vi "Virbmain.vi"(0 "Channel 4":T9={" frequency 1"=20, "signal type 1"=enum."Sine Wave", "amplitude 1"=2.0, "offset"=0.0, "phase"=0.0} {"phase" format="%.2p"; "offset" format="%0.2p"; "amplitude 1" format="%0.2p"}, 1 "Channel 3":T9={" frequency 1"=20, "signal type 1"=enum."Sine Wave", "amplitude 1"=2.0, "offset"=0.0, "phase"=0.0} {"phase" format="%.2p"; "offset" format="%0.2p"; "amplitude 1" format="%0.2p"}, 2 "Channel 2":T9={" frequency 1"=20, "signal type 1"=enum."Sine Wave", "amplitude 1"=2.0, "offset"=0.0, "phase"=0.0} {"phase" format="%.2p"; "offset" format="%0.2p"; "amplitude 1" format="%0.2p"}, 3 "Channel 1":T9={" frequency 1"=20, "signal type 1"=enum."Sine Wave", "amplitude 1"=2.0, "offset"=0.0, "phase"=0.0} {"phase" format="%.2p"; "offset" format="%0.2p"; "amplitude 1" format="%0.2p"}, 4 "Time(ms)":i32, 5 "Model List":i32(listbox), 6 "Play Button":bool, 7 "Project Name":string, 9 "OK Button":bool, 10 "Remove Project":bool, 11 "Add Project":bool) -> ()   [LabVIEW 2015]
uses:
  Typedef/Test_State.ctl
  Typedef/State.ctl
  Typedef/Data.ctl
  Typedef/Timer State.ctl
  <vilib>/Utility/xml.llb/Read From XML File(string).vi
  <vilib>/Utility/xml.llb/Write to XML File(string).vi
  <vilib>/measure/NI_MABase.lvlib
panel:
  out "TCP connect":bool
  in  "Right":T1={"Channel 1"={" frequency 1"=25, "signal type 1"=enum."Sine Wave", "amplitude 1"=2.0, "offset"=0.0, "phase"=0.0}, "Channel 2"={" frequency 1"=0, "signal type 1"=enum."Sine Wave", "amplitude 1"=0, "offset"=0.0, "phase"=0.0}, "Channel 3"={" frequency 1"=25, "signal type 1"=enum."Sine Wave", "amplitude 1"=2.0, "offset"=0.0, "phase"=0}, "Channel 4"={" frequency 1"=25, "signal type 1"=enum."Sine Wave", "amplitude 1"=2.0, "offset"=0.0, "phase"=0}}
  in  "Back":T2={"Channel 1"={" frequency 1"=0, "signal type 1"=enum."Sine Wave", "amplitude 1"=0, "offset"=0.0, "phase"=0.0}, "Channel 2"={" frequency 1"=25, "signal type 1"=enum."Sine Wave", "amplitude 1"=2.0, "offset"=0.0, "phase"=0.0}, "Channel 3"={" frequency 1"=25, "signal type 1"=enum."Sine Wave", "amplitude 1"=2.0, "offset"=0, "phase"=0}, "Channel 4"={" frequency 1"=25, "signal type 1"=enum."Sine Wave", "amplitude 1"=2.0, "offset"=0.0, "phase"=0}}
  in  "Left":T3={"Channel 1"={" frequency 1"=25, "signal type 1"=enum."Sine Wave", "amplitude 1"=2.0, "offset"=0, "phase"=0.0}, "Channel 2"={" frequency 1"=25, "signal type 1"=enum."Sine Wave", "amplitude 1"=2.0, "offset"=0, "phase"=0}, "Channel 3"={" frequency 1"=25, "signal type 1"=enum."Sine Wave", "amplitude 1"=2.0, "offset"=0, "phase"=0}, "Channel 4"={" frequency 1"=0, "signal type 1"=enum."Sine Wave", "amplitude 1"=0, "offset"=0, "phase"=0.0}}
  in  "Front":T4={"Channel 1"={" frequency 1"=25, "signal type 1"=enum."Sine Wave", "amplitude 1"=2.0, "offset"=0.0, "phase"=0.0}, "Channel 2"={" frequency 1"=25, "signal type 1"=enum."Sine Wave", "amplitude 1"=2.0, "offset"=0.0, "phase"=0}, "Channel 3"={" frequency 1"=0, "signal type 1"=enum."Sine Wave", "amplitude 1"=0, "offset"=0.0, "phase"=0.0}, "Channel 4"={" frequency 1"=25, "signal type 1"=enum."Sine Wave", "amplitude 1"=2.0, "offset"=0.0, "phase"=0}}
  in  "Center":T5={"Channel 1"={" frequency 1"=25, "signal type 1"=enum."Sine Wave", "amplitude 1"=1.25, "offset"=0, "phase"=0.0}, "Channel 2"={" frequency 1"=25, "signal type 1"=enum."Sine Wave", "amplitude 1"=1.25, "offset"=0, "phase"=90}, "Channel 3"={" frequency 1"=25, "signal type 1"=enum."Sine Wave", "amplitude 1"=1.25, "offset"=0, "phase"=180}, "Channel 4"={" frequency 1"=25, "signal type 1"=enum."Sine Wave", "amplitude 1"=1.25, "offset"=0, "phase"=270}}
  in  "Bump":T6={"Channel 1"={" frequency 1"=25, "signal type 1"=enum."Sine Wave", "amplitude 1"=2.0, "offset"=0, "phase"=0.0}, "Channel 2"={" frequency 1"=25, "signal type 1"=enum."Sine Wave", "amplitude 1"=2.0, "offset"=0, "phase"=0.0}, "Channel 3"={" frequency 1"=25, "signal type 1"=enum."Sine Wave", "amplitude 1"=2.0, "offset"=0, "phase"=0.0}, "Channel 4"={" frequency 1"=25, "signal type 1"=enum."Sine Wave", "amplitude 1"=2.0, "offset"=0, "phase"=0.0}}
  out "Test State":T7
  out "Testing?":bool
  out "Test Setting":waveform(dbl)[](array[waveform])
  out "DataTable":T8(array[cluster])
  in  "Tab Control":enum32{"Main", "Project", "Set"}(tab)
  in  "Setting(Main)":bool
  in  "Project(Main)":bool
  out "Running":bool
  out "Channel 4 Wave (Main)":waveform(dbl)(graph)
  out "Channel 3 Wave (Main)":waveform(dbl)(graph)
  out "Channel 2 Wave (Main)":waveform(dbl)(graph)
  out "Channel 1 Wave (Main)":waveform(dbl)(graph)
  in  "Stop Button":bool
  in  "Center":bool
  in  "Bump":bool
  in  "Rightward":bool
  in  "Leftward":bool
  in  "Backward":bool
  in  "Frontward":bool
  out "Project":string
  in  "Exit Button":bool
  in  "Project List":i32(listbox)
  in  "Main(Project)":bool
  in  "Setting(Project)":bool
  out "Test Time":dbl
  in  "Save Button":bool
  in  "Remove":bool
  in  "Add":bool
  out "Channel 4 Wave":waveform(dbl)(graph)
  out "Channel 3 Wave":waveform(dbl)(graph)
  out "Channel 2 Wave":waveform(dbl)(graph)
  out "Channel 1 Wave":waveform(dbl)(graph)
  out "Testing":bool
  in  "Project(Setting)":bool
  in  "Main(Setting)":bool
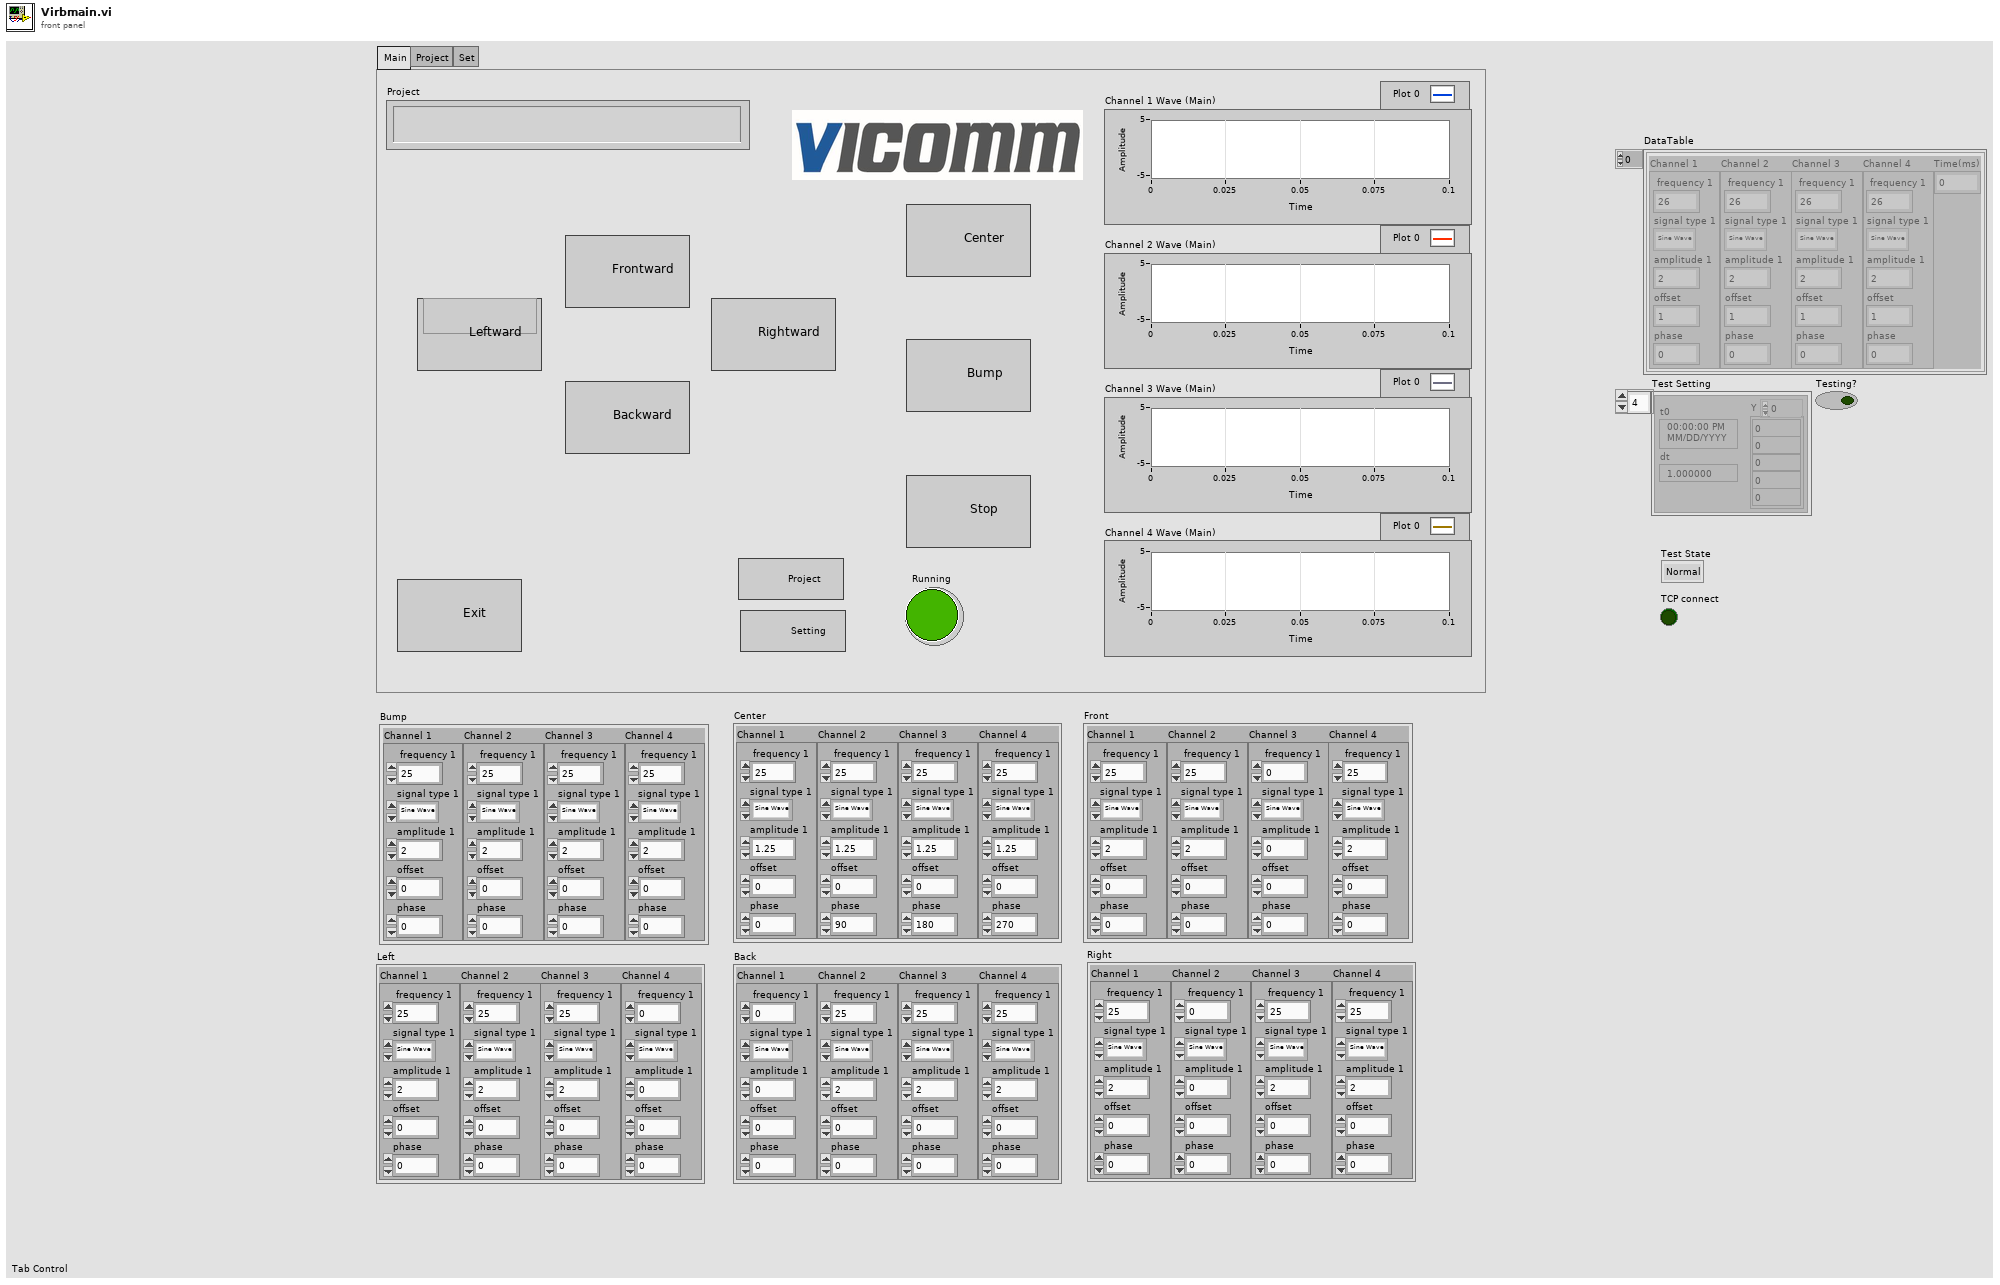
[diagram p1: front panel]
types:
  T1 = cluster{"Channel 1":cluster{" frequency 1":i32, "signal type 1":enum16{"Sine Wave", "Triangle Wave", "Square Wave", "Sawtooth Wave"}, "amplitude 1":dbl, "offset":dbl, "phase":dbl}, "Channel 2":cluster{" frequency 1":i32, "signal type 1":enum16{"Sine Wave", "Triangle Wave", "Square Wave", "Sawtooth Wave"}, "amplitude 1":i32, "offset":dbl, "phase":dbl}, "Channel 3":cluster{" frequency 1":i32, "signal type 1":enum16{"Sine Wave", "Triangle Wave", "Square Wave", "Sawtooth Wave"}, "amplitude 1":dbl, "offset":dbl, "phase":i32}, "Channel 4":cluster{" frequency 1":i32, "signal type 1":enum16{"Sine Wave", "Triangle Wave", "Square Wave", "Sawtooth Wave"}, "amplitude 1":dbl, "offset":dbl, "phase":i32}}
  T2 = cluster{"Channel 1":cluster{" frequency 1":i32, "signal type 1":enum16{"Sine Wave", "Triangle Wave", "Square Wave", "Sawtooth Wave"}, "amplitude 1":i32, "offset":dbl, "phase":dbl}, "Channel 2":cluster{" frequency 1":i32, "signal type 1":enum16{"Sine Wave", "Triangle Wave", "Square Wave", "Sawtooth Wave"}, "amplitude 1":dbl, "offset":dbl, "phase":dbl}, "Channel 3":cluster{" frequency 1":i32, "signal type 1":enum16{"Sine Wave", "Triangle Wave", "Square Wave", "Sawtooth Wave"}, "amplitude 1":dbl, "offset":i32, "phase":i32}, "Channel 4":cluster{" frequency 1":i32, "signal type 1":enum16{"Sine Wave", "Triangle Wave", "Square Wave", "Sawtooth Wave"}, "amplitude 1":dbl, "offset":dbl, "phase":i32}}
  T3 = cluster{"Channel 1":cluster{" frequency 1":i32, "signal type 1":enum16{"Sine Wave", "Triangle Wave", "Square Wave", "Sawtooth Wave"}, "amplitude 1":dbl, "offset":i32, "phase":dbl}, "Channel 2":cluster{" frequency 1":i32, "signal type 1":enum16{"Sine Wave", "Triangle Wave", "Square Wave", "Sawtooth Wave"}, "amplitude 1":dbl, "offset":i32, "phase":i32}, "Channel 3":cluster{" frequency 1":i32, "signal type 1":enum16{"Sine Wave", "Triangle Wave", "Square Wave", "Sawtooth Wave"}, "amplitude 1":dbl, "offset":i32, "phase":i32}, "Channel 4":cluster{" frequency 1":i32, "signal type 1":enum16{"Sine Wave", "Triangle Wave", "Square Wave", "Sawtooth Wave"}, "amplitude 1":i32, "offset":i32, "phase":dbl}}
  T4 = cluster{"Channel 1":cluster{" frequency 1":i32, "signal type 1":enum16{"Sine Wave", "Triangle Wave", "Square Wave", "Sawtooth Wave"}, "amplitude 1":dbl, "offset":dbl, "phase":dbl}, "Channel 2":cluster{" frequency 1":i32, "signal type 1":enum16{"Sine Wave", "Triangle Wave", "Square Wave", "Sawtooth Wave"}, "amplitude 1":dbl, "offset":dbl, "phase":i32}, "Channel 3":cluster{" frequency 1":i32, "signal type 1":enum16{"Sine Wave", "Triangle Wave", "Square Wave", "Sawtooth Wave"}, "amplitude 1":i32, "offset":dbl, "phase":dbl}, "Channel 4":cluster{" frequency 1":i32, "signal type 1":enum16{"Sine Wave", "Triangle Wave", "Square Wave", "Sawtooth Wave"}, "amplitude 1":dbl, "offset":dbl, "phase":i32}}
  T5 = cluster{"Channel 1":cluster{" frequency 1":i32, "signal type 1":enum16{"Sine Wave", "Triangle Wave", "Square Wave", "Sawtooth Wave"}, "amplitude 1":dbl, "offset":i32, "phase":dbl}, "Channel 2":cluster{" frequency 1":i32, "signal type 1":enum16{"Sine Wave", "Triangle Wave", "Square Wave", "Sawtooth Wave"}, "amplitude 1":dbl, "offset":i32, "phase":i32}, "Channel 3":cluster{" frequency 1":i32, "signal type 1":enum16{"Sine Wave", "Triangle Wave", "Square Wave", "Sawtooth Wave"}, "amplitude 1":dbl, "offset":i32, "phase":i32}, "Channel 4":cluster{" frequency 1":i32, "signal type 1":enum16{"Sine Wave", "Triangle Wave", "Square Wave", "Sawtooth Wave"}, "amplitude 1":dbl, "offset":i32, "phase":i32}}
  T6 = cluster{"Channel 1":cluster{" frequency 1":i32, "signal type 1":enum16{"Sine Wave", "Triangle Wave", "Square Wave", "Sawtooth Wave"}, "amplitude 1":dbl, "offset":i32, "phase":dbl}, "Channel 2":cluster{" frequency 1":i32, "signal type 1":enum16{"Sine Wave", "Triangle Wave", "Square Wave", "Sawtooth Wave"}, "amplitude 1":dbl, "offset":i32, "phase":dbl}, "Channel 3":cluster{" frequency 1":i32, "signal type 1":enum16{"Sine Wave", "Triangle Wave", "Square Wave", "Sawtooth Wave"}, "amplitude 1":dbl, "offset":i32, "phase":dbl}, "Channel 4":cluster{" frequency 1":i32, "signal type 1":enum16{"Sine Wave", "Triangle Wave", "Square Wave", "Sawtooth Wave"}, "amplitude 1":dbl, "offset":i32, "phase":dbl}}
  T7 = typedef "Test_State.ctl" = enum16{"Normal", "Bump", "Center"}
  T8 = cluster{"Channel 1":cluster{" frequency 1":u32, "signal type 1":enum16{"Sine Wave", "Triangle Wave", "Square Wave", "Sawtooth Wave"}, "amplitude 1":dbl, "offset":dbl, "phase":dbl}, "Channel 2":cluster{" frequency 1":u32, "signal type 1":enum16{"Sine Wave", "Triangle Wave", "Square Wave", "Sawtooth Wave"}, "amplitude 1":dbl, "offset":dbl, "phase":dbl}, "Channel 3":cluster{" frequency 1":u32, "signal type 1":enum16{"Sine Wave", "Triangle Wave", "Square Wave", "Sawtooth Wave"}, "amplitude 1":dbl, "offset":dbl, "phase":dbl}, "Channel 4":cluster{" frequency 1":u32, "signal type 1":enum16{"Sine Wave", "Triangle Wave", "Square Wave", "Sawtooth Wave"}, "amplitude 1":dbl, "offset":dbl, "phase":dbl}, "Time(ms)":i32}[]
  T9 = cluster{" frequency 1":u32, "signal type 1":enum16{"Sine Wave", "Triangle Wave", "Square Wave", "Sawtooth Wave"}, "amplitude 1":dbl, "offset":dbl, "phase":dbl}
  T10 = typedef "Data.ctl" = cluster{"Channel Table":cluster{"Channel 1":cluster{" frequency 1":u32, "signal type 1":enum16{"Sine Wave", "Triangle Wave", "Square Wave", "Sawtooth Wave"}, "amplitude 1":dbl, "offset":dbl, "phase":dbl}, "Channel 2":cluster{" frequency 1":u32, "signal type 1":enum16{"Sine Wave", "Triangle Wave", "Square Wave", "Sawtooth Wave"}, "amplitude 1":dbl, "offset":dbl, "phase":dbl}, "Channel 3":cluster{" frequency 1":u32, "signal type 1":enum16{"Sine Wave", "Triangle Wave", "Square Wave", "Sawtooth Wave"}, "amplitude 1":dbl, "offset":dbl, "phase":dbl}, "Channel 4":cluster{" frequency 1":u32, "signal type 1":enum16{"Sine Wave", "Triangle Wave", "Square Wave", "Sawtooth Wave"}, "amplitude 1":dbl, "offset":dbl, "phase":dbl}, "Time(ms)":i32}[], "Model List name":string[], "Channel 1 Wave":waveform(dbl), "Channel 2 Wave":waveform(dbl), "Channel 3 Wave":waveform(dbl), "Channel 4 Wave":waveform(dbl), "Testing":bool, "Set Time":i32, "Elapse Time":dbl, "Channel 1":cluster{" frequency 1":u32, "signal type 1":enum16{"Sine Wave", "Triangle Wave", "Square Wave", "Sawtooth Wave"}, "amplitude 1":dbl, "offset":dbl, "phase":dbl}, "Channel 2":cluster{" frequency 1":u32, "signal type 1":enum16{"Sine Wave", "Triangle Wave", "Square Wave", "Sawtooth Wave"}, "amplitude 1":dbl, "offset":dbl, "phase":dbl}, "Channel 3":cluster{" frequency 1":u32, "signal type 1":enum16{"Sine Wave", "Triangle Wave", "Square Wave", "Sawtooth Wave"}, "amplitude 1":dbl, "offset":dbl, "phase":dbl}, "Channel 4":cluster{" frequency 1":u32, "signal type 1":enum16{"Sine Wave", "Triangle Wave", "Square Wave", "Sawtooth Wave"}, "amplitude 1":dbl, "offset":dbl, "phase":dbl}, "ModelList Num":i32, "Stop":bool, "Button":bool, "Button Time":i32, "Elapsed ?":bool, "Channel 1 Wave (Main)":waveform(dbl), "Channel 2 Wave (Main)":waveform(dbl), "Channel 3 Wave (Main)":waveform(dbl), "Channel 4 Wave (Main)":waveform(dbl), "Project List name":string[], "Project Name":string, "Project Path":path, "ProjectList Num":i32, "Project Name(Set)":string}
  T11 = enum16{"Standard", "Buffered", "CRLF", "Immediate"}
  T12 = typedef "State.ctl" = enum16{"Initalize", "Idle", "Update", "Channel1", "Channel2", "Channel3", "Channel4", "ModelList", "Add", "Remove", "Set Time", "Test", "Start Time", "Check Time", "Save", "Frontward", "Leftward", "Backward", "Rightward", "Stop", "Center", "Bump", "Add Project", "Remove Project", "Project List", "Project Name", "Project OK", "Exit"}
  T13 = typedef "Timer State.ctl" = enum16{"Start", "Check"}
  T14 = cluster{"State":T12, "Channel 1":cluster{" frequency 1":u32, "signal type 1":enum16{"Sine Wave", "Triangle Wave", "Square Wave", "Sawtooth Wave"}, "amplitude 1":dbl, "offset":dbl, "phase":dbl}}
  T15 = cluster{"State":T12, "Channel 2":cluster{" frequency 1":u32, "signal type 1":enum16{"Sine Wave", "Triangle Wave", "Square Wave", "Sawtooth Wave"}, "amplitude 1":dbl, "offset":dbl, "phase":dbl}}
  T16 = cluster{"State":T12, "Channel 3":cluster{" frequency 1":u32, "signal type 1":enum16{"Sine Wave", "Triangle Wave", "Square Wave", "Sawtooth Wave"}, "amplitude 1":dbl, "offset":dbl, "phase":dbl}}
  T17 = cluster{"State":T12, "Channel 4":cluster{" frequency 1":u32, "signal type 1":enum16{"Sine Wave", "Triangle Wave", "Square Wave", "Sawtooth Wave"}, "amplitude 1":dbl, "offset":dbl, "phase":dbl}}
  T18 = cluster{"DataTable":cluster{"Channel 1":cluster{" frequency 1":u32, "signal type 1":enum16{"Sine Wave", "Triangle Wave", "Square Wave", "Sawtooth Wave"}, "amplitude 1":dbl, "offset":dbl, "phase":dbl}, "Channel 2":cluster{" frequency 1":u32, "signal type 1":enum16{"Sine Wave", "Triangle Wave", "Square Wave", "Sawtooth Wave"}, "amplitude 1":dbl, "offset":dbl, "phase":dbl}, "Channel 3":cluster{" frequency 1":u32, "signal type 1":enum16{"Sine Wave", "Triangle Wave", "Square Wave", "Sawtooth Wave"}, "amplitude 1":dbl, "offset":dbl, "phase":dbl}, "Channel 4":cluster{" frequency 1":u32, "signal type 1":enum16{"Sine Wave", "Triangle Wave", "Square Wave", "Sawtooth Wave"}, "amplitude 1":dbl, "offset":dbl, "phase":dbl}, "Time(ms)":i32}[], "Item Names":string[]}
  T19 = enum16{"Sine Wave", "Triangle Wave", "Square Wave", "Sawtooth Wave"}
  T20 = cluster{"Channel 1":cluster{" frequency 1":u32, "signal type 1":enum16{"Sine Wave", "Triangle Wave", "Square Wave", "Sawtooth Wave"}, "amplitude 1":dbl, "offset":dbl, "phase":dbl}, "Channel 2":cluster{" frequency 1":u32, "signal type 1":enum16{"Sine Wave", "Triangle Wave", "Square Wave", "Sawtooth Wave"}, "amplitude 1":dbl, "offset":dbl, "phase":dbl}, "Channel 3":cluster{" frequency 1":u32, "signal type 1":enum16{"Sine Wave", "Triangle Wave", "Square Wave", "Sawtooth Wave"}, "amplitude 1":dbl, "offset":dbl, "phase":dbl}, "Channel 4":cluster{" frequency 1":u32, "signal type 1":enum16{"Sine Wave", "Triangle Wave", "Square Wave", "Sawtooth Wave"}, "amplitude 1":dbl, "offset":dbl, "phase":dbl}, "Time(ms)":i32}
  T21 = cluster{" frequency 1":u32, "signal type 1":enum16{"Sine Wave", "Triangle Wave", "Square Wave", "Sawtooth Wave"}, "amplitude 1":dbl, "offset":dbl, "phase":dbl}[]
  T22 = cluster{"Channel 1":cluster{" frequency 1":u32, "signal type 1":enum16{"Sine Wave", "Triangle Wave", "Square Wave", "Sawtooth Wave"}, "amplitude 1":dbl, "offset":dbl, "phase":dbl}, "Channel 2":cluster{" frequency 1":u32, "signal type 1":enum16{"Sine Wave", "Triangle Wave", "Square Wave", "Sawtooth Wave"}, "amplitude 1":dbl, "offset":dbl, "phase":dbl}, "Channel 3":cluster{" frequency 1":u32, "signal type 1":enum16{"Sine Wave", "Triangle Wave", "Square Wave", "Sawtooth Wave"}, "amplitude 1":dbl, "offset":dbl, "phase":dbl}, "Channel 4":cluster{" frequency 1":u32, "signal type 1":enum16{"Sine Wave", "Triangle Wave", "Square Wave", "Sawtooth Wave"}, "amplitude 1":dbl, "offset":dbl, "phase":dbl}, "Set Time":i32}
  T23 = cluster{"Channel 1":cluster{" frequency 1":u32, "signal type 1":enum16{"Sine Wave", "Triangle Wave", "Square Wave", "Sawtooth Wave"}, "amplitude 1":dbl, "offset":dbl, "phase":dbl}, "Channel 2":cluster{" frequency 1":u32, "signal type 1":enum16{"Sine Wave", "Triangle Wave", "Square Wave", "Sawtooth Wave"}, "amplitude 1":dbl, "offset":dbl, "phase":dbl}, "Channel 3":cluster{" frequency 1":u32, "signal type 1":enum16{"Sine Wave", "Triangle Wave", "Square Wave", "Sawtooth Wave"}, "amplitude 1":dbl, "offset":dbl, "phase":dbl}, "Channel 4":cluster{" frequency 1":u32, "signal type 1":enum16{"Sine Wave", "Triangle Wave", "Square Wave", "Sawtooth Wave"}, "amplitude 1":dbl, "offset":dbl, "phase":dbl}, "Set Time":i32}[]
  T24 = cluster{"Channel Table":cluster{"Channel 1":cluster{" frequency 1":u32, "signal type 1":enum16{"Sine Wave", "Triangle Wave", "Square Wave", "Sawtooth Wave"}, "amplitude 1":dbl, "offset":dbl, "phase":dbl}, "Channel 2":cluster{" frequency 1":u32, "signal type 1":enum16{"Sine Wave", "Triangle Wave", "Square Wave", "Sawtooth Wave"}, "amplitude 1":dbl, "offset":dbl, "phase":dbl}, "Channel 3":cluster{" frequency 1":u32, "signal type 1":enum16{"Sine Wave", "Triangle Wave", "Square Wave", "Sawtooth Wave"}, "amplitude 1":dbl, "offset":dbl, "phase":dbl}, "Channel 4":cluster{" frequency 1":u32, "signal type 1":enum16{"Sine Wave", "Triangle Wave", "Square Wave", "Sawtooth Wave"}, "amplitude 1":dbl, "offset":dbl, "phase":dbl}, "Time(ms)":i32}[], "Model List name":string[]}
  T25 = cluster{" frequency 1":i32, "signal type 1":enum16{"Sine Wave", "Triangle Wave", "Square Wave", "Sawtooth Wave"}, "amplitude 1":dbl, "offset":dbl, "phase":dbl}
  T26 = cluster{" frequency 1":i32, "signal type 1":enum16{"Sine Wave", "Triangle Wave", "Square Wave", "Sawtooth Wave"}, "amplitude 1":dbl, "offset":dbl, "phase":i32}
  T27 = cluster{" frequency 1":i32, "signal type 1":enum16{"Sine Wave", "Triangle Wave", "Square Wave", "Sawtooth Wave"}, "amplitude 1":i32, "offset":dbl, "phase":dbl}
  T28 = cluster{" frequency 1":i32, "signal type 1":enum16{"Sine Wave", "Triangle Wave", "Square Wave", "Sawtooth Wave"}, "amplitude 1":dbl, "offset":dbl, "phase":dbl}[]
  T29 = cluster{" frequency 1":i32, "signal type 1":enum16{"Sine Wave", "Triangle Wave", "Square Wave", "Sawtooth Wave"}, "amplitude 1":dbl, "offset":i32, "phase":dbl}
  T30 = cluster{" frequency 1":i32, "signal type 1":enum16{"Sine Wave", "Triangle Wave", "Square Wave", "Sawtooth Wave"}, "amplitude 1":dbl, "offset":i32, "phase":i32}
  T31 = cluster{" frequency 1":i32, "signal type 1":enum16{"Sine Wave", "Triangle Wave", "Square Wave", "Sawtooth Wave"}, "amplitude 1":i32, "offset":i32, "phase":dbl}
  T32 = cluster{" frequency 1":i32, "signal type 1":enum16{"Sine Wave", "Triangle Wave", "Square Wave", "Sawtooth Wave"}, "amplitude 1":dbl, "offset":i32, "phase":dbl}[]
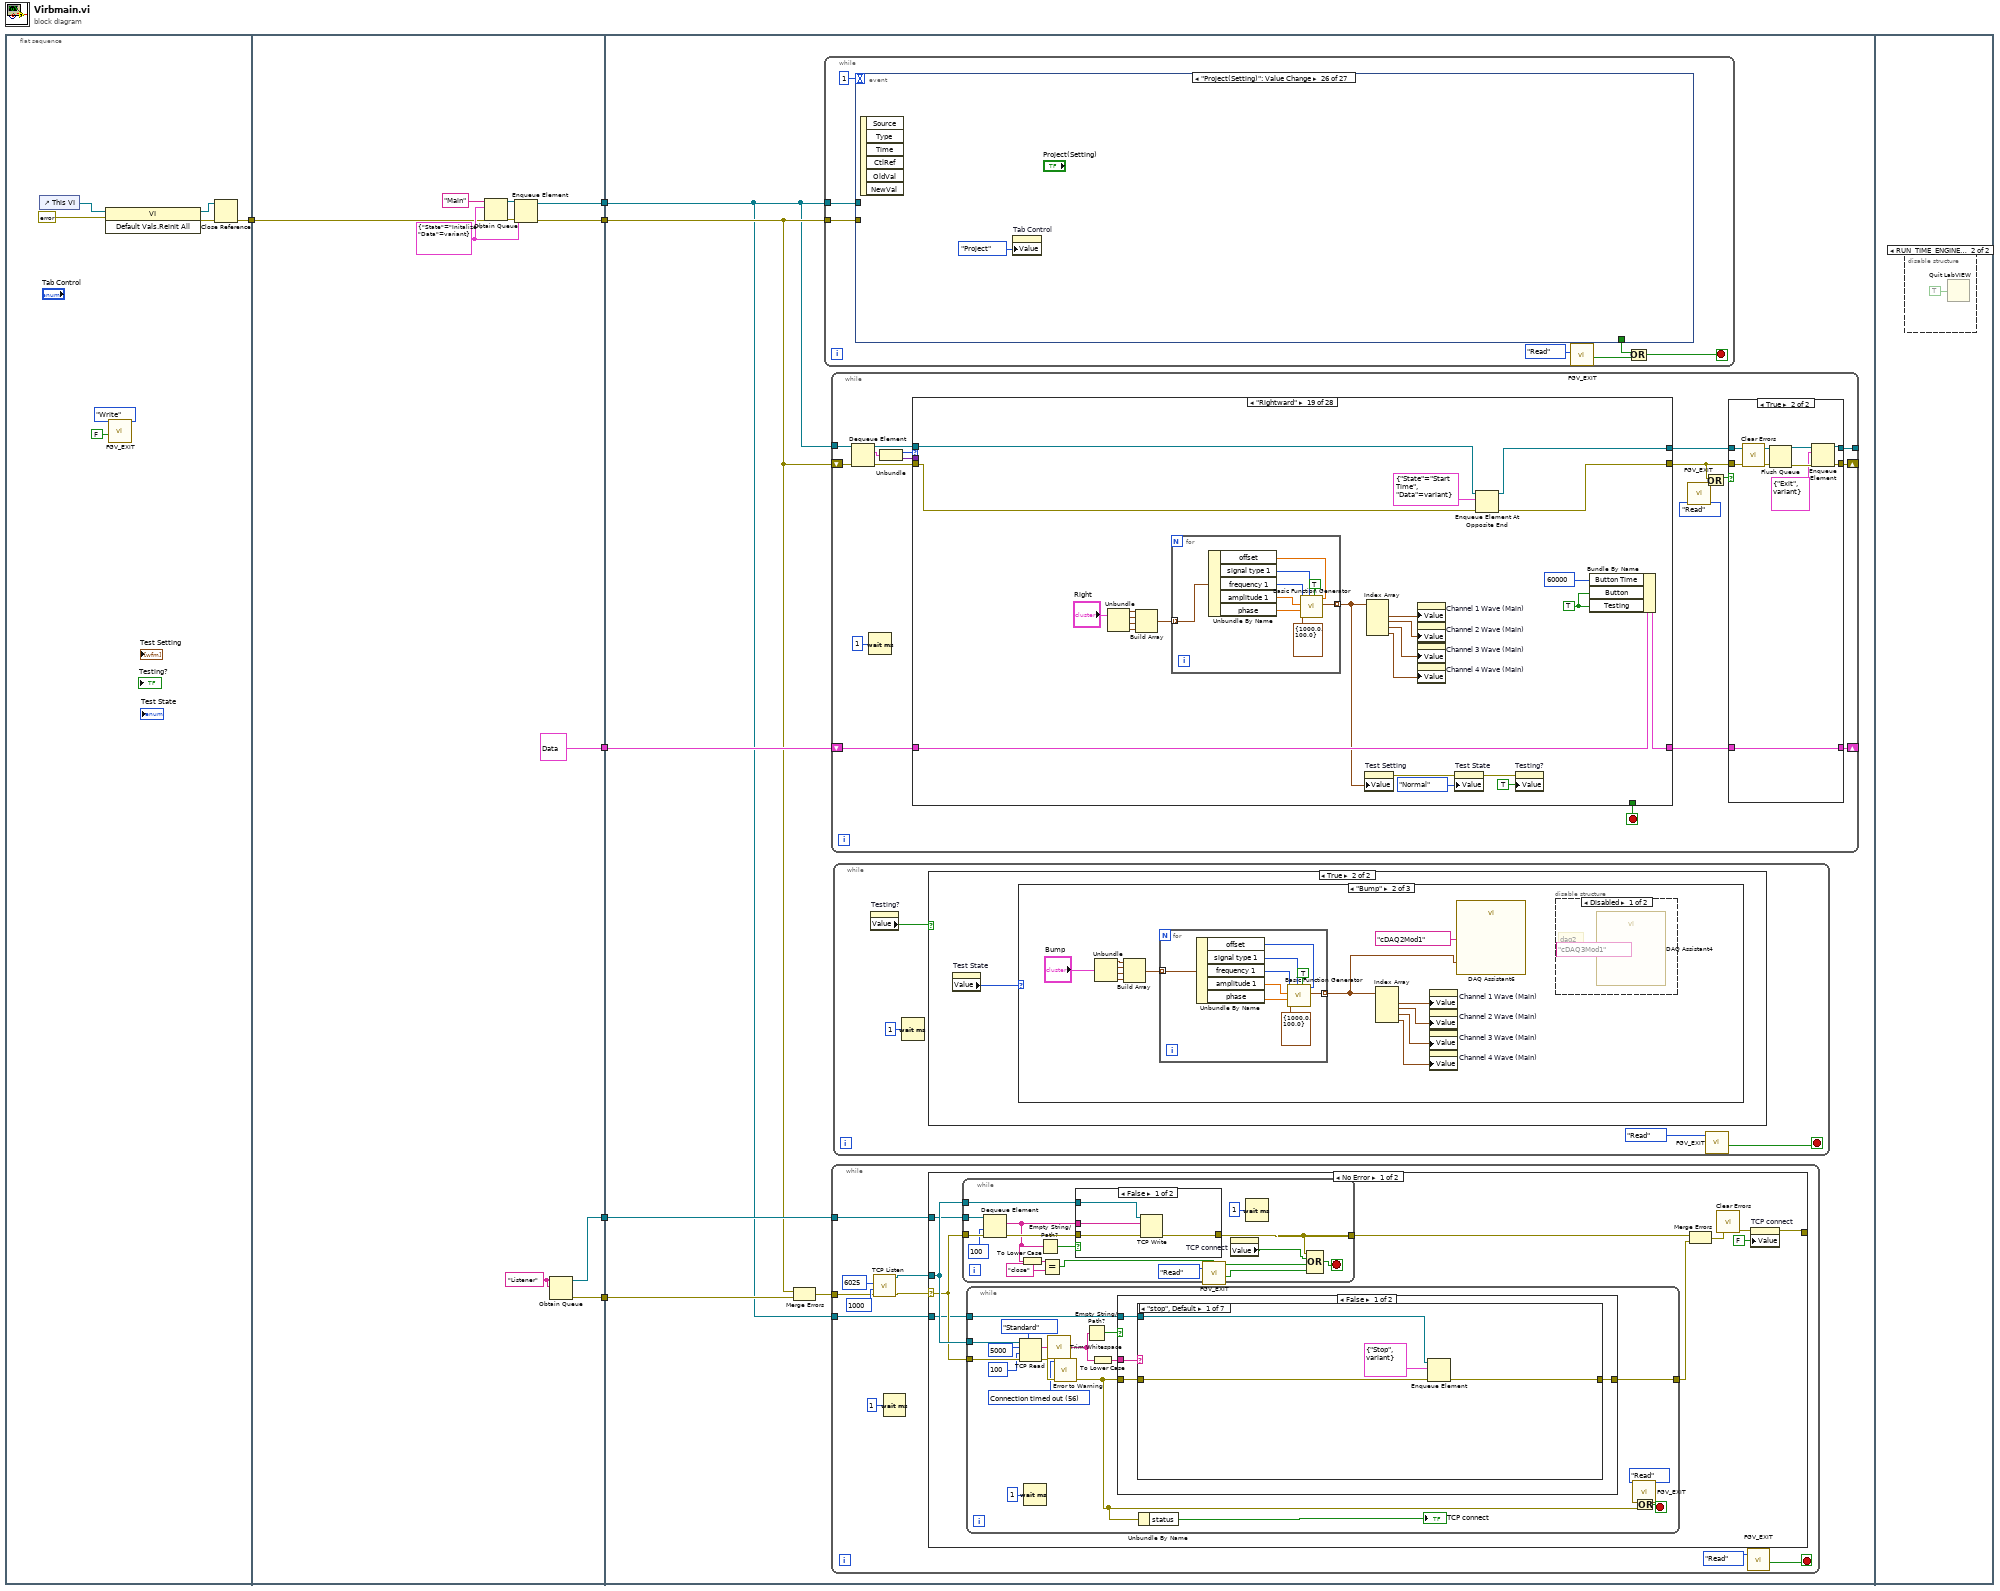
[diagram p0: block diagram]
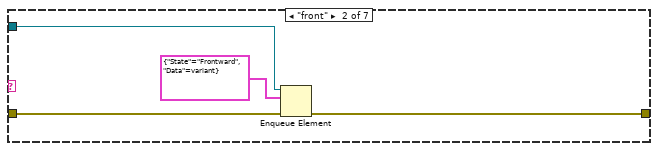
[diagram p2: hidden frame]
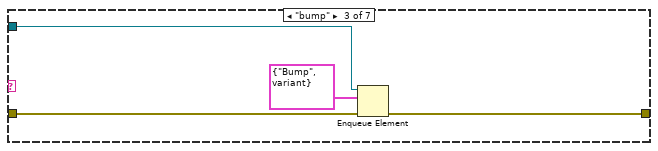
[diagram p3: hidden frame]
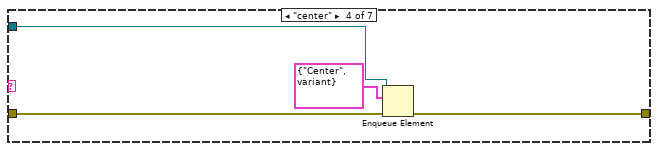
[diagram p4: hidden frame]
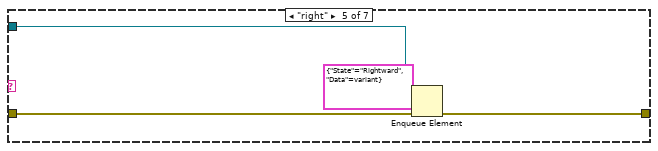
[diagram p5: hidden frame]
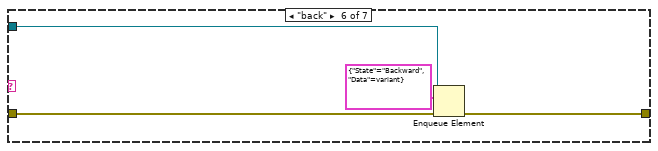
[diagram p6: hidden frame]
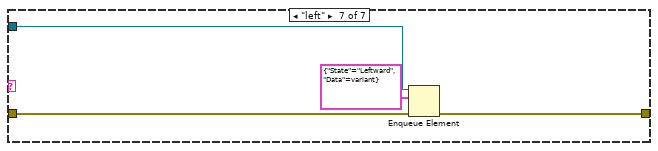
[diagram p7: hidden frame]
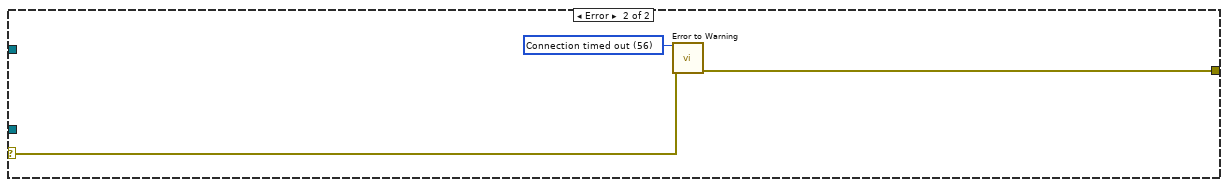
[diagram p10: hidden frame]
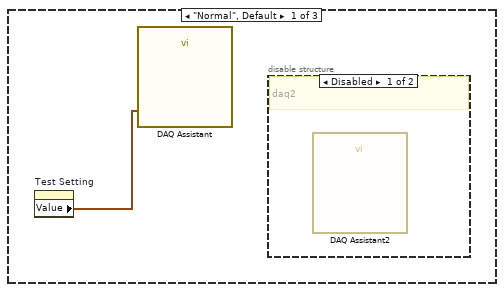
[diagram p12: hidden frame]
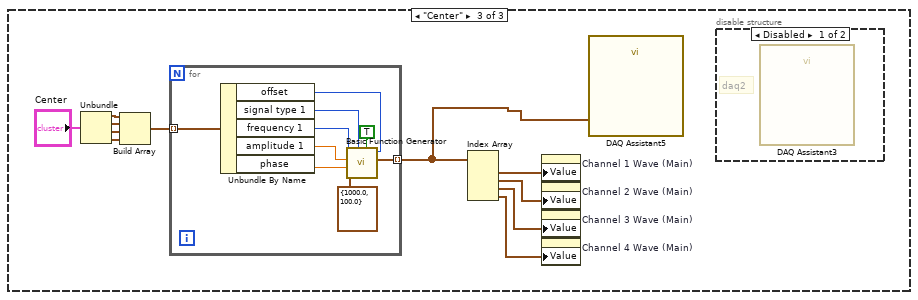
[diagram p15: hidden frame]
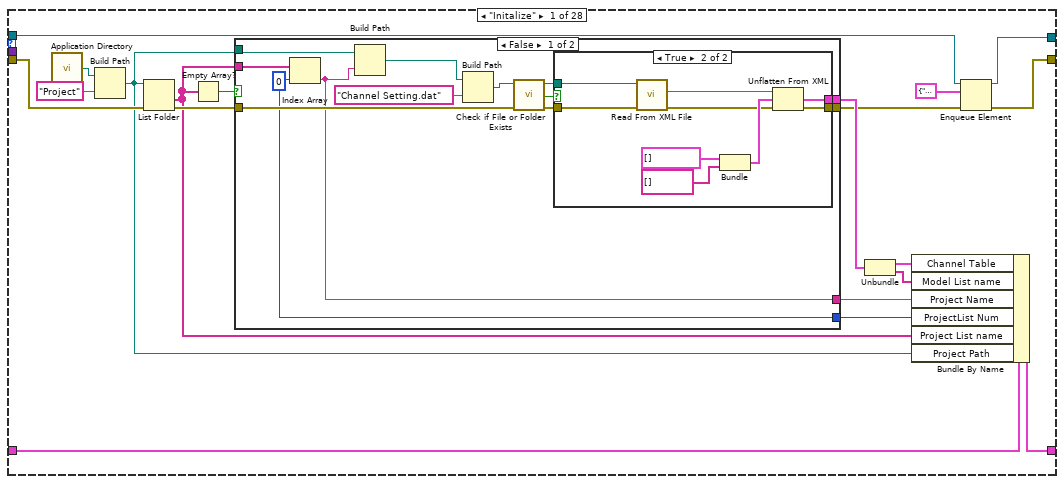
[diagram p18: hidden frame]
diagram:
  n1 = flat-sequence {
    tunnel: [w10] -> w3
    tunnel: [w20] -> w6
    tunnel: [w19] -> w5
    tunnel: [T10 {"Channel Table"=[], "Model List name"=[], "Channel 1 Wave"={"t0"=timestamp(0 s since 1904-01-01), "dt"=1.0, "Y"=[]}, "Channel 2 Wave"={"t0"=timestamp(0 s since 1904-01-01), "dt"=1.0, "Y"=[]}, "Channel 3 Wave"={"t0"=timestamp(0 s since 1904-01-01), "dt"=1.0, "Y"=[]}, "Channel 4 Wave"={"t0"=timestamp(0 s since 1904-01-01), "dt"=1.0, "Y"=[]}, "Testing"=FALSE, "Set Time"=0, "Elapse Time"=0.0, "Channel 1"={" frequency 1"=20, "signal type 1"=enum."Sine Wave", "amplitude 1"=2.0, "offset"=0.0, "phase"=0.0}, "Channel 2"={" frequency 1"=20, "signal type 1"=enum."Sine Wave", "amplitude 1"=2.0, "offset"=0.0, "phase"=0.0}, "Channel 3"={" frequency 1"=20, "signal type 1"=enum."Sine Wave", "amplitude 1"=2.0, "offset"=0.0, "phase"=0.0}, "Channel 4"={" frequency 1"=20, "signal type 1"=enum."Sine Wave", "amplitude 1"=2.0, "offset"=0.0, "phase"=0.0}, "ModelList Num"=0, "Stop"=FALSE, "Button"=FALSE, "Button Time"=0, "Elapsed ?"=FALSE, "Channel 1 Wave (Main)"={"t0"=timestamp(0 s since 1904-01-01), "dt"=1.0, "Y"=[]}, "Channel 2 Wave (Main)"={"t0"=timestamp(0 s since 1904-01-01), "dt"=1.0, "Y"=[]}, "Channel 3 Wave (Main)"={"t0"=timestamp(0 s since 1904-01-01), "dt"=1.0, "Y"=[]}, "Channel 4 Wave (Main)"={"t0"=timestamp(0 s since 1904-01-01), "dt"=1.0, "Y"=[]}, "Project List name"=[], "Project Name"="", "Project Path"=path "", "ProjectList Num"=0, "Project Name(Set)"=""}] -> w4
    tunnel: w3 -> [w17]
    tunnel: [w15] -> w2
    tunnel: [w14] -> w1
    tunnel: w6 -> [w25]
    tunnel: w5 -> [w26]
    tunnel: w4 -> [w30]
    tunnel: w2 -> [w29]
    tunnel: w1 -> [w28]
    frame #0 {
      n2 = control-ref of="This VI"() -> (w13:refnum<vi>)
      n3 = invoke class="VI" method="Default Vals.Reinit All"(reference=w13, error in=errorcluster {"status"=FALSE, "code"=0, "source"=""} ("error in (no error)")) -> (reference out=w11:refnum<vi>, error out=w12:errorcluster)  [unwired: 1 in, 1 out]
      n4 = call "FGV_EXIT.vi"("Function"=enum16{"Read", "Write"}."Write", "EXIT"=FALSE) -> ()  [unwired: 6 in, 1 out]
      n5 = Close Reference(reference=w11, error in (no error)=w12) -> (error out=w10:errorcluster)
    }
    frame #1 {
      w16 = "Listener" ("name (unnamed)")
      w21 = cluster{"State":T12, "Data":variant} {"State"=enum."Initalize", "Data"=variant}
      n6 = Obtain Queue(name (unnamed)="Main", element data type=w21, error in (no error)=w17) -> (queue out=w23:refnum<queue>, error out=w24:errorcluster)  [unwired: 2 in, 1 out]
      n7 = Enqueue Element(queue=w23, element=w21, error in (no error)=w24) -> (queue out=w20:refnum<queue>, error out=w19:errorcluster)  [unwired: 1 in, 1 out]
      n8 = Obtain Queue(name (unnamed)=w16, element data type=w16) -> (queue out=w15:refnum<queue>, error out=w14:errorcluster)  [unwired: 3 in, 1 out]
    }
    frame #2 {
      n9 = Merge Errors(w26, w28) -> (w27:errorcluster)
      n10 = while {
        tunnel: w25 -> [w818]
        tunnel: w26 -> [w817]
        stop <- w815 stop-if-true
        n11 = event shown="[25] \"Project(Setting)\": Value Change" {
          selector: _ -> [_ _ _ _ _ _ _ _ _ _ _ _ _ _ _ _ _ _ _ _ _ _ _ _ _ _ _]
          dyn-events: _ -> [_ _ _ _ _ _ _ _ _ _ _ _ _ _ _ _ _ _ _ _ _ _ _ _ _ _ _]
          timeout: 1 -> [_ _ _ _ _ _ _ _ _ _ _ _ _ _ _ _ _ _ _ _ _ _ _ _ _ _ _]
          tunnel: [_ w821 _ _ _ _ _ _ _ _ _ _ _ _ _ _ _ _ _ _ _ _ _ _ _ _ _] -> w819
          tunnel: w818 -> [_ w825 w829 w834 w840 w872 w875 w878 w881 w884 w887 w890 w893 w896 w899 w902 w905 w910 w915 w919 w921 _ _ _ _ _ _]
          tunnel: w817 -> [_ w826 w828 w835 w839 w873 w876 w879 w882 w885 w888 w891 w894 w897 w900 w903 w906 w911 w916 w918 w922 _ _ _ _ _ _]
          event Timeout {
            n12 = event-data() -> ()  [unwired: 1 in, 3 out]
          }
          event "Exit Button": Value Change {
            w821 = TRUE
            n13 = event-data() -> ()  [unwired: 1 in, 2 out]
            n14 = Flush Queue(queue=w825, error in (no error)=w826) -> (queue out=w823:refnum<queue>, error out=w824:errorcluster)  [unwired: 1 out]
            n15 = Enqueue Element(queue=w823, element=cluster{"State":T12, "Data":variant} {"State"=enum."Exit", "Data"=variant}, error in (no error)=w824) -> ()  [unwired: 1 in, 3 out]
            n16 = call "FGV_EXIT.vi"("Function"=enum16{"Read", "Write"}."Write", "EXIT"=w821) -> ()  [unwired: 6 in, 1 out]
          }
          event "Play Button": Value Change {
            n17 = event-data() -> ()  [unwired: 1 in, 6 out]
            n18 = Enqueue Element(queue=w829, element=cluster{"State":T12, "Data":variant} {"State"=enum."Test", "Data"=variant}, error in (no error)=w828) -> ()  [unwired: 1 in, 3 out]
          }
          event "Time(ms)": Value Change {
            n19 = event-data() -> ()  [unwired: 1 in, 1 out]
            n20 = Bundle(cluster=cluster{"State":T12, "Data":variant} {"State"=enum."Initalize", "Data"=variant}, "State"=State."Set Time", "Data"="Time(ms)") -> (w832:cluster{"State":T12, "Data":variant})
            n21 = Enqueue Element(queue=w834, element=w832, error in (no error)=w835) -> ()  [unwired: 1 in, 3 out]
          }
          event "Channel 1", "Channel 2", "Channel 4", "Channel 3": Value Change {
            n22 = event-data() -> ("CtlRef"=w845:refnum<vi>)  [unwired: 1 in]
            n23 = property class="Clust (strict)"(reference=w845) -> ("Label.Text"=w844:string)  [unwired: 1 in, 2 out]
            n24 = Match Pattern(string=w844, regular expression="Channel") -> (after substring=w842:string)  [unwired: 1 in, 3 out]
            n25 = Decimal String To Number(string=w842) -> (number=w841:i32)  [unwired: 2 in, 1 out]
            n26 = case shown="4" w841 {
              tunnel: w840 -> [w848 w852 w857 w862 w867]
              tunnel: w839 -> [w847 w853 w858 w863 w868]
              tunnel: [w847 w853 w858 w863 w868] -> w838
              tunnel: [w848 w852 w857 w862 w867] -> w837
              tunnel: [cluster{"State":T12, "Data":variant} {"State"=enum."Update", "Data"=variant} w850 w856 w860 w866] -> w836
              frame 0, Default {
              }
              frame 1 {
                n27 = Bundle("State"=State."Channel1", "Channel 1"="Channel 1") -> (w850:T14)  [unwired: 1 in]
              }
              frame 2 {
                n28 = Bundle("State"=State."Channel2", "Channel 2"="Channel 2") -> (w856:T15)  [unwired: 1 in]
              }
              frame 3 {
                n29 = Bundle("State"=State."Channel3", "Channel 3"="Channel 3") -> (w860:T16)  [unwired: 1 in]
              }
              frame 4 {
                n30 = Bundle("State"=State."Channel4", "Channel 4"="Channel 4") -> (w866:T17)  [unwired: 1 in]
              }
            }
            n31 = Enqueue Element(queue=w837, element=w836, error in (no error)=w838) -> ()  [unwired: 1 in, 3 out]
          }
          event "Model List": Value Change {
            n32 = event-data() -> ("NewVal"=w869:i32)  [unwired: 1 in]
            n33 = Bundle By Name(cluster=cluster{"State":T12, "Data":variant} {"State"=enum."ModelList", "Data"=variant}, "Data"=w869) -> (w871:cluster{"State":T12, "Data":variant})
            n34 = Enqueue Element(queue=w872, element=w871, error in (no error)=w873) -> ()  [unwired: 1 in, 3 out]
          }
          event "Add": Value Change {
            n35 = event-data() -> ()  [unwired: 1 in, 1 out]
            n36 = Enqueue Element(queue=w875, element=cluster{"State":T12, "Data":variant} {"State"=enum."Add", "Data"=variant}, error in (no error)=w876) -> ()  [unwired: 1 in, 3 out]
          }
          event "Remove": Value Change {
            n37 = event-data() -> ()  [unwired: 1 in, 2 out]
            n38 = Enqueue Element(queue=w878, element=cluster{"State":T12, "Data":variant} {"State"=enum."Remove", "Data"=variant}, error in (no error)=w879) -> ()  [unwired: 1 in, 3 out]
          }
          event "Save Button": Value Change {
            n39 = event-data() -> ()  [unwired: 1 in, 2 out]
            n40 = Enqueue Element(queue=w881, element=cluster{"State":T12, "Data":variant} {"State"=enum."Save", "Data"=variant}, error in (no error)=w882) -> ()  [unwired: 1 in, 3 out]
          }
          event "Frontward": Value Change {
            n41 = event-data() -> ()  [unwired: 1 in, 2 out]
            n42 = Enqueue Element(queue=w884, element=cluster{"State":T12, "Data":variant} {"State"=enum."Frontward", "Data"=variant}, error in (no error)=w885) -> ()  [unwired: 1 in, 3 out]
          }
          event "Leftward": Value Change {
            n43 = event-data() -> ()  [unwired: 1 in, 2 out]
            n44 = Enqueue Element(queue=w887, element=cluster{"State":T12, "Data":variant} {"State"=enum."Leftward", "Data"=variant}, error in (no error)=w888) -> ()  [unwired: 1 in, 3 out]
          }
          event "Backward": Value Change {
            n45 = event-data() -> ()  [unwired: 1 in, 2 out]
            n46 = Enqueue Element(queue=w890, element=cluster{"State":T12, "Data":variant} {"State"=enum."Backward", "Data"=variant}, error in (no error)=w891) -> ()  [unwired: 1 in, 3 out]
          }
          event "Rightward": Value Change {
            n47 = event-data() -> ()  [unwired: 1 in, 2 out]
            n48 = Enqueue Element(queue=w893, element=cluster{"State":T12, "Data":variant} {"State"=enum."Rightward", "Data"=variant}, error in (no error)=w894) -> ()  [unwired: 1 in, 3 out]
          }
          event "Center": Value Change {
            n49 = event-data() -> ()  [unwired: 1 in, 6 out]
            n50 = Enqueue Element(queue=w896, element=cluster{"State":T12, "Data":variant} {"State"=enum."Center", "Data"=variant}, error in (no error)=w897) -> ()  [unwired: 1 in, 3 out]
          }
          event "Bump": Value Change {
            n51 = event-data() -> ()  [unwired: 1 in, 6 out]
            n52 = Enqueue Element(queue=w899, element=cluster{"State":T12, "Data":variant} {"State"=enum."Bump", "Data"=variant}, error in (no error)=w900) -> ()  [unwired: 1 in, 3 out]
          }
          event "Add Project": Value Change {
            n53 = event-data() -> ()  [unwired: 1 in, 6 out]
            n54 = Enqueue Element(queue=w902, element=cluster{"State":T12, "Data":variant} {"State"=enum."Add Project", "Data"=variant}, error in (no error)=w903) -> ()  [unwired: 1 in, 3 out]
          }
          event "Remove Project": Value Change {
            n55 = event-data() -> ()  [unwired: 1 in, 6 out]
            n56 = Enqueue Element(queue=w905, element=cluster{"State":T12, "Data":variant} {"State"=enum."Remove Project", "Data"=variant}, error in (no error)=w906) -> ()  [unwired: 1 in, 3 out]
          }
          event "Project Name": Value Change {
            n57 = event-data() -> ("NewVal"=w907:string)  [unwired: 1 in]
            n58 = Bundle By Name(cluster=cluster{"State":T12, "Data":variant} {"State"=enum."Project Name", "Data"=variant}, "Data"=w907) -> (w908:cluster{"State":T12, "Data":variant})
            n59 = Enqueue Element(queue=w910, element=w908, error in (no error)=w911) -> ()  [unwired: 1 in, 3 out]
          }
          event "Project List": Value Change {
            n60 = event-data() -> ("NewVal"=w912:i32)  [unwired: 1 in, 5 out]
            n61 = Bundle By Name(cluster=cluster{"State":T12, "Data":variant} {"State"=enum."Project List", "Data"=variant}, "Data"=w912) -> (w913:cluster{"State":T12, "Data":variant})
            n62 = Enqueue Element(queue=w915, element=w913, error in (no error)=w916) -> ()  [unwired: 1 in, 3 out]
          }
          event "OK Button": Value Change {
            n63 = event-data() -> ()  [unwired: 1 in, 6 out]
            n64 = Enqueue Element(queue=w919, element=cluster{"State":T12, "Data":variant} {"State"=enum."Project OK", "Data"=variant}, error in (no error)=w918) -> ()  [unwired: 1 in, 3 out]
          }
          event "Stop Button": Value Change {
            n65 = event-data() -> ()  [unwired: 1 in, 2 out]
            n66 = Enqueue Element(queue=w921, element=cluster{"State":T12, "Data":variant} {"State"=enum."Stop", "Data"=variant}, error in (no error)=w922) -> ()  [unwired: 1 in, 3 out]
          }
          event "Project(Main)": Value Change {
            n67 = event-data() -> ()  [unwired: 1 in, 6 out]
            n68 = property on="Tab Control" class="TabCtl (strict)"("Value"=enum32{"Main", "Project", "Set"}."Project" ("Tab Control")) -> ()  [unwired: 2 in, 2 out]
          }
          event "Setting(Main)": Value Change {
            n69 = event-data() -> ()  [unwired: 1 in, 6 out]
            n70 = property on="Tab Control" class="TabCtl (strict)"("Value"=enum32{"Main", "Project", "Set"}."Set" ("Tab Control")) -> ()  [unwired: 2 in, 2 out]
          }
          event "Main(Project)": Value Change {
            n71 = event-data() -> ()  [unwired: 1 in, 6 out]
            n72 = property on="Tab Control" class="TabCtl (strict)"("Value"=enum32{"Main", "Project", "Set"}."Main" ("Tab Control")) -> ()  [unwired: 2 in, 2 out]
          }
          event "Setting(Project)": Value Change {
            n73 = event-data() -> ()  [unwired: 1 in, 6 out]
            n74 = property on="Tab Control" class="TabCtl (strict)"("Value"=enum32{"Main", "Project", "Set"}."Set" ("Tab Control")) -> ()  [unwired: 2 in, 2 out]
          }
          event "Project(Setting)": Value Change {
            n75 = event-data() -> ()  [unwired: 1 in, 6 out]
            n76 = property on="Tab Control" class="TabCtl (strict)"("Value"=enum32{"Main", "Project", "Set"}."Project" ("Tab Control")) -> ()  [unwired: 2 in, 2 out]
          }
          event "Main(Setting)": Value Change {
            n77 = event-data() -> ()  [unwired: 1 in, 6 out]
            n78 = property on="Tab Control" class="TabCtl (strict)"("Value"=enum32{"Main", "Project", "Set"}."Main" ("Tab Control")) -> ()  [unwired: 2 in, 2 out]
          }
        }
        n79 = call "FGV_EXIT.vi"("Function"=enum16{"Read", "Write"}."Read") -> ("EXIT out"=w813:bool)  [unwired: 7 in]
        n80 = Or(x=w819, y=w813) -> (x .or. y?=w815:bool)
      }
      n81 = while {
        tunnel: w25 -> [w193]
        shift-right: [w184] -> _
        shift-left: w30 -> [w187]
        tunnel: [w183] -> _
        shift-right: [w182] -> _
        shift-left: w26 -> [w192]
        stop <- w180 stop-if-true
        n82 = Dequeue Element(queue=w193, error in (no error)=w192) -> (queue out=w191:refnum<queue>, element=w189:cluster{"State":T12, "Data":variant}, error out=w190:errorcluster)  [unwired: 1 in, 1 out]
        n83 = Wait (ms)(milliseconds to wait=u32 1) -> ()  [unwired: 1 out]
        n84 = Unbundle(w189) -> ("State"=w188:T12, "Data"=w181:variant)
        n85 = case shown="\"Rightward\"" w188 {
          tunnel: w191 -> [w218 w261 w296 w323 w343 w363 w383 w388 w446 w460 w466 w482 w499 w510 w521 w552 w585 w618 w651 w669 w680 w692 w705 w744 w755 w766 w778 w810]
          tunnel: w190 -> [w213 w259 w298 w320 w340 w360 w368 w411 w424 w457 w469 w484 w500 w511 w520 w549 w582 w615 w648 w667 w679 w691 w702 w741 w747 w758 w771 w811]
          tunnel: w187 -> [w223 w254 w286 w318 w338 w358 w380 w407 w437 w451 w465 w479 w492 w507 w522 w547 w580 w613 w646 w664 w676 w688 w699 w739 w751 w762 w773 w812]
          tunnel: [w222 w257 w286 w317 w337 w357 w379 w406 w435 w450 w464 w487 w496 w506 w522 w546 w579 w612 w645 w663 w675 w687 w698 w738 w750 w761 w774 w812] -> w185
          tunnel: [w217 w260 w295 w321 w341 w361 w381 w387 w445 w459 w466 w481 w498 w509 w521 w551 w584 w617 w650 w668 w677 w689 w704 w743 w754 w765 w777 w810] -> w186
          tunnel: [w215 w258 w297 w322 w342 w362 w382 w389 w423 w458 w462 w483 w497 w508 w520 w548 w581 w614 w647 w666 w678 w690 w701 w740 w752 w763 w775 w811] -> w175
          tunnel: w181 -> [_ _ _ w319 w339 w359 w367 w412 _ _ w468 _ _ _ _ _ _ _ _ _ _ _ _ _ w748 w759 _ _]
          tunnel: [_ _ _ _ _ _ _ _ _ _ _ _ _ _ _ _ _ _ _ _ _ _ _ _ _ _ _ w809] -> w180
          frame "Initalize" {
            n86 = call <vilib>:"Application Directory.vi"() -> ("Application Directory"=w214:path)
            n87 = Build Path(base path=w214, name or relative path="Project") -> (appended path=w209:path)
            n88 = List Folder(path=w209, error in=w213) -> (folder names=w207:string[], error out=w212:errorcluster)  [unwired: 2 in, 2 out]
            n89 = Empty Array?(array=w207) -> (empty?=w206:bool)
            n90 = case shown="False" w206 {
              tunnel: [w236 _] -> w224
              tunnel: [w235 w248] -> w219
              tunnel: w212 -> [w230 w248]
              tunnel: w207 -> [w228 _]
              tunnel: [w227 _] -> w210
              tunnel: w209 -> [w226 _]
              tunnel: [w225 _] -> w208
              frame False {
                w225 = 0
                n91 = Index Array(array=w228, index=w225) -> (element=w227:string)
                n92 = Build Path(base path=w226, name or relative path=w227) -> (appended path=w229:path)
                n93 = Build Path(base path=w229, name or relative path="Channel Setting.dat") -> (appended path=w233:path)
                n94 = call <vilib>:"Check if File or Folder Exists.vi"("error in (no error)"=w230, "path"=w233) -> ("error out"=w234:errorcluster, "file or folder exists?"=w232:bool, "dup path"=w231:path)  [unwired: 7 in]
                n95 = case shown="True" w232 {
                  tunnel: [_ w242] -> w236
                  tunnel: [w238 w241] -> w235
                  tunnel: w234 -> [w238 w240]
                  tunnel: w231 -> [_ w239]
                  frame False {
                  }
                  frame True {
                    n96 = call-poly <vilib>:"Read From XML File.vi"("error in (no error)"=w240, "XML File Path"=w239) -> ("error out"=w243:errorcluster, "XML Elements"=w247:string)  [unwired: 7 in, 1 out]
                    n97 = Bundle("DataTable"=T8 [], "Item Names"=string[] []) -> (w244:T18)  [unwired: 1 in]
                    n98 = Unflatten From XML(xml string=w247, type=w244, error in (no error)=w243) -> (value=w242:T18, error out=w241:errorcluster)
                  }
                }
              }
              frame True {
              }
            }
            n99 = Unbundle(w224) -> ("DataTable"=w221:T8, "Item Names"=w220:string[])
            n100 = Bundle By Name(cluster=w223, "Channel Table"=w221, "Model List name"=w220, "Project Name"=w210, "ProjectList Num"=w208, "Project List name"=w207, "Project Path"=w209) -> (w222:T10)
            n101 = Enqueue Element(queue=w218, element=cluster{"State":T12, "Data":variant} {"State"=enum."Update", "Data"=variant}, error in (no error)=w219) -> (queue out=w217:refnum<queue>, error out=w215:errorcluster)  [unwired: 1 in, 1 out]
          }
          frame "Idle", Default {
            n102 = Unbundle By Name(w254) -> ("Stop"=w251:bool, "Testing"=w255:bool, "Elapsed ?"=w250:bool)
            n103 = Not(x=w251) -> (.not. x?=w252:bool)
            n104 = Not(x=w250) -> (.not. x?=w256:bool)
            n105 = Compound Arithmetic op=AND(w252, w255, w256) -> (w249:bool)
            "Testing" <- w249
            "Running" <- w249
            n106 = Bundle By Name(cluster=w254, "Testing"=w249) -> (w253:T10)
            n107 = case shown="False" w249 {
              tunnel: w261 -> [w266 w280]
              tunnel: [w265 w279] -> w260
              tunnel: w259 -> [w264 w277]
              tunnel: [w263 w281] -> w258
              tunnel: w253 -> [w268 w278]
              tunnel: [w267 w278] -> w257
              tunnel: w251 -> [w262 _]
              frame False {
                n108 = case shown="False" w262 {
                  tunnel: w268 -> [w269 w274]
                  tunnel: [w269 w273] -> w267
                  tunnel: w266 -> [w271 w276]
                  tunnel: [w271 w276] -> w265
                  tunnel: w264 -> [w270 w275]
                  tunnel: [w270 w275] -> w263
                  frame False {
                  }
                  frame True {
                    n109 = Bundle By Name(cluster=w274, "Stop"=FALSE) -> (w273:T10)
                  }
                }
              }
              frame True {
                n110 = Enqueue Element(queue=w280, element=cluster{"State":T12, "Data":variant} {"State"=enum."Check Time", "Data"=variant}, error in (no error)=w277) -> (queue out=w279:refnum<queue>, error out=w281:errorcluster)  [unwired: 1 in, 1 out]
              }
            }
          }
          frame "Update" {
            n111 = Unbundle By Name(w286) -> ("Project Name"=→"Project":string, "Elapse Time"=→"Test Time":dbl, "Channel 1 Wave"=→"Channel 1 Wave":waveform(dbl), "Channel 2 Wave"=→"Channel 2 Wave":waveform(dbl), "Channel 3 Wave"=→"Channel 3 Wave":waveform(dbl), "Channel 4 Wave"=→"Channel 4 Wave":waveform(dbl), "Channel Table"=→"DataTable":T8, "Model List name"=w302:string[], "Channel 1"=w293:T9, "Channel 2"=w292:T9, "Channel 3"=w291:T9, "Channel 4"=w290:T9, "Set Time"=w289:i32, "Project List name"=w285:string[], "Project Name(Set)"=w283:string)
            n112 = property on="Model List" class="LstBox (strict)"("Item Names"=w302) -> ()  [unwired: 2 in, 2 out]
            n113 = property on="Channel 1" class="Clust (strict)"("Value"=w293) -> ()  [unwired: 2 in, 2 out]
            n114 = property on="Channel 2" class="Clust (strict)"("Value"=w292) -> ()  [unwired: 2 in, 2 out]
            n115 = property on="Channel 3" class="Clust (strict)"("Value"=w291) -> ()  [unwired: 2 in, 2 out]
            n116 = property on="Channel 4" class="Clust (strict)"("Value"=w290) -> ()  [unwired: 2 in, 2 out]
            n117 = property on="Time(ms)" class="DigNum (strict)"("Value"=w289) -> ()  [unwired: 2 in, 2 out]
            n118 = property on="Project List" class="LstBox (strict)"("Item Names"=w285) -> ()  [unwired: 2 in, 2 out]
            n119 = property on="Project Name" class="Str"("Value"=w283) -> ()  [unwired: 2 in, 2 out]
            n120 = Enqueue Element(queue=w296, element=cluster{"State":T12, "Data":variant} {"State"=enum."Idle", "Data"=variant}, error in (no error)=w298) -> (queue out=w295:refnum<queue>, error out=w297:errorcluster)  [unwired: 1 in, 1 out]
          }
          frame "Channel1" {
            n121 = Variant To Data(error in=w320, type=T9 {" frequency 1"=20, "signal type 1"=enum."Sine Wave", "amplitude 1"=2.0, "offset"=0.0, "phase"=0.0} ("Channel 2"), Variant=w319) -> (data=w304:T9, error out=w312:errorcluster)
            n122 = Unbundle By Name(w304) -> ("offset"=w306:dbl, "signal type 1"=w307:T19, "frequency 1"=w308:u32, "amplitude 1"=w309:dbl, "phase"=w310:dbl)
            n123 = call <vilib>:"Basic Function Generator.vi"("offset"=w306, "reset signal"=TRUE, "sampling info"=cluster{"Fs":dbl, "#s":dbl} {"Fs"=1000.0, "#s"=100.0} ("sampling info 4"), "signal type"=w307, "error in (no error)"=w312, "phase"=w310, "amplitude"=w309, "frequency"=w308) -> ("error out"=w311:errorcluster, "signal out"=w305:waveform(dbl))  [unwired: 1 in, 1 out]
            n124 = Bundle By Name(cluster=w318, "Channel 1 Wave"=w305, "Channel 1"=w304) -> (w317:T10)
            n125 = Enqueue Element At Opposite End(queue=w323, element=cluster{"State":T12, "Data":variant} {"State"=enum."Update", "Data"=variant}, error in (no error)=w311) -> (queue out=w321:refnum<queue>, error out=w322:errorcluster)  [unwired: 1 in, 1 out]
          }
          frame "Channel2" {
            n126 = Variant To Data(error in=w340, type=T9 {" frequency 1"=20, "signal type 1"=enum."Sine Wave", "amplitude 1"=2.0, "offset"=0.0, "phase"=0.0} ("Channel 2"), Variant=w339) -> (data=w324:T9, error out=w328:errorcluster)
            n127 = Unbundle By Name(w324) -> ("offset"=w329:dbl, "signal type 1"=w330:T19, "frequency 1"=w331:u32, "amplitude 1"=w332:dbl, "phase"=w333:dbl)
            n128 = call <vilib>:"Basic Function Generator.vi"("offset"=w329, "reset signal"=TRUE, "sampling info"=cluster{"Fs":dbl, "#s":dbl} {"Fs"=1000.0, "#s"=100.0} ("sampling info 4"), "signal type"=w330, "error in (no error)"=w328, "phase"=w333, "amplitude"=w332, "frequency"=w331) -> ("error out"=w327:errorcluster, "signal out"=w326:waveform(dbl))  [unwired: 1 in, 1 out]
            n129 = Bundle By Name(cluster=w338, "Channel 2 Wave"=w326, "Channel 2"=w324) -> (w337:T10)
            n130 = Enqueue Element At Opposite End(queue=w343, element=cluster{"State":T12, "Data":variant} {"State"=enum."Update", "Data"=variant}, error in (no error)=w327) -> (queue out=w341:refnum<queue>, error out=w342:errorcluster)  [unwired: 1 in, 1 out]
          }
          frame "Channel3" {
            n131 = Variant To Data(error in=w360, type=T9 {" frequency 1"=20, "signal type 1"=enum."Sine Wave", "amplitude 1"=2.0, "offset"=0.0, "phase"=0.0} ("Channel 2"), Variant=w359) -> (data=w345:T9, error out=w348:errorcluster)
            n132 = Unbundle By Name(w345) -> ("offset"=w349:dbl, "signal type 1"=w350:T19, "frequency 1"=w351:u32, "amplitude 1"=w352:dbl, "phase"=w353:dbl)
            n133 = call <vilib>:"Basic Function Generator.vi"("offset"=w349, "reset signal"=TRUE, "sampling info"=cluster{"Fs":dbl, "#s":dbl} {"Fs"=1000.0, "#s"=100.0} ("sampling info 4"), "signal type"=w350, "error in (no error)"=w348, "phase"=w353, "amplitude"=w352, "frequency"=w351) -> ("error out"=w347:errorcluster, "signal out"=w344:waveform(dbl))  [unwired: 1 in, 1 out]
            n134 = Bundle By Name(cluster=w358, "Channel 3 Wave"=w344, "Channel 3"=w345) -> (w357:T10)
            n135 = Enqueue Element At Opposite End(queue=w363, element=cluster{"State":T12, "Data":variant} {"State"=enum."Update", "Data"=variant}, error in (no error)=w347) -> (queue out=w361:refnum<queue>, error out=w362:errorcluster)  [unwired: 1 in, 1 out]
          }
          frame "Channel4" {
            n136 = Variant To Data(error in=w368, type=T9 {" frequency 1"=20, "signal type 1"=enum."Sine Wave", "amplitude 1"=2.0, "offset"=0.0, "phase"=0.0} ("Channel 2"), Variant=w367) -> (data=w364:T9, error out=w370:errorcluster)
            n137 = Unbundle By Name(w364) -> ("offset"=w371:dbl, "signal type 1"=w372:T19, "frequency 1"=w373:u32, "amplitude 1"=w374:dbl, "phase"=w375:dbl)
            n138 = call <vilib>:"Basic Function Generator.vi"("offset"=w371, "reset signal"=TRUE, "sampling info"=cluster{"Fs":dbl, "#s":dbl} {"Fs"=1000.0, "#s"=100.0} ("sampling info 4"), "signal type"=w372, "error in (no error)"=w370, "phase"=w375, "amplitude"=w374, "frequency"=w373) -> ("error out"=w366:errorcluster, "signal out"=w365:waveform(dbl))  [unwired: 1 in, 1 out]
            n139 = Bundle By Name(cluster=w380, "Channel 4 Wave"=w365, "Channel 4"=w364) -> (w379:T10)
            n140 = Enqueue Element At Opposite End(queue=w383, element=cluster{"State":T12, "Data":variant} {"State"=enum."Update", "Data"=variant}, error in (no error)=w366) -> (queue out=w381:refnum<queue>, error out=w382:errorcluster)  [unwired: 1 in, 1 out]
          }
          frame "ModelList" {
            n141 = Unbundle By Name(w407) -> ("Channel Table"=w409:T8)
            n142 = Variant To Data(error in=w411, type=0, Variant=w412) -> (data=w385:i32, error out=w390:errorcluster)
            n143 = Index Array(array=w409, index=w385) -> (element=w408:T20)
            n144 = Unbundle(w408) -> ("Channel 1"=w404:T9, "Channel 2"=w403:T9, "Channel 3"=w402:T9, "Channel 4"=w401:T9, "Time(ms)"=w405:i32)
            n145 = Build Array(w404, w403, w402, w401) -> (w400:T21)
            n146 = for {
              tunnel: w400 -> [w413] mode=indexing
              tunnel: [w414] -> w384 mode=indexing
              tunnel: [w413] -> w399 mode=indexing
              n147 = Unbundle By Name(w413) -> ("offset"=w415:dbl, "signal type 1"=w416:T19, "frequency 1"=w417:u32, "amplitude 1"=w418:dbl, "phase"=w419:dbl)
              n148 = call <vilib>:"Basic Function Generator.vi"("offset"=w415, "reset signal"=TRUE, "sampling info"=cluster{"Fs":dbl, "#s":dbl} {"Fs"=1000.0, "#s"=100.0} ("sampling info 4"), "signal type"=w416, "phase"=w419, "amplitude"=w418, "frequency"=w417) -> ("signal out"=w414:waveform(dbl))  [unwired: 2 in, 2 out]
            }
            n149 = Index Array(array=w399) -> (element #1=w398:T9, element #2=w393:T9, element #3=w392:T9, element #4=w391:T9)  [unwired: 4 in]
            n150 = Index Array(array=w384) -> (element #1=w397:waveform(dbl), element #2=w396:waveform(dbl), element #3=w395:waveform(dbl), element #4=w394:waveform(dbl))  [unwired: 4 in]
            n151 = Bundle By Name(cluster=w407, "Channel 1 Wave"=w397, "Channel 2 Wave"=w396, "Channel 3 Wave"=w395, "Channel 4 Wave"=w394, "Channel 1"=w398, "Channel 2"=w393, "Channel 3"=w392, "Channel 4"=w391, "Set Time"=w405, "ModelList Num"=w385) -> (w406:T10)
            n152 = Enqueue Element At Opposite End(queue=w388, element=cluster{"State":T12, "Data":variant} {"State"=enum."Update", "Data"=variant}, error in (no error)=w390) -> (queue out=w387:refnum<queue>, error out=w389:errorcluster)  [unwired: 1 in, 1 out]
          }
          frame "Add" {
            n153 = Unbundle By Name(w437) -> ("Channel Table"=w444:T8, "Channel 1"=w443:T9, "Channel 2"=w442:T9, "Channel 3"=w441:T9, "Channel 4"=w440:T9, "Set Time"=w439:i32, "Model List name"=w426:string[])
            n154 = Array Size(array=w426) -> (size(s)=w429:i32)
            n155 = Bundle("Channel 1"=w443, "Channel 2"=w442, "Channel 3"=w441, "Channel 4"=w440, "Set Time"=w439) -> (w438:T22)  [unwired: 1 in]
            n156 = Decrement(x=w429) -> (x-1=w434:i32)
            n157 = Index Array(array=w426, index=w434) -> (element=w430:string)
            n158 = Build Array (concatenate)(w444, w438) -> (w436:T23)
            n159 = Match Pattern(string=w430, regular expression="Model") -> (after substring=w432:string)  [unwired: 1 in, 3 out]
            n160 = Decimal String To Number(string=w432) -> (number=w428:i32)  [unwired: 2 in, 1 out]
            n161 = Increment(x=w428) -> (x+1=w422:i32)
            n162 = Format Into String(format string="Model%d", w422) -> (resulting string=w427:string)  [unwired: 2 in, 1 out]
            n163 = Build Array (concatenate)(w426, w427) -> (w425:string[])
            n164 = Bundle By Name(cluster=w437, "Channel Table"=w436, "Model List name"=w425) -> (w435:T10)
            n165 = Enqueue Element At Opposite End(queue=w446, element=cluster{"State":T12, "Data":variant} {"State"=enum."Update", "Data"=variant}, error in (no error)=w424) -> (queue out=w445:refnum<queue>, error out=w423:errorcluster)  [unwired: 1 in, 1 out]
          }
          frame "Remove" {
            n166 = Unbundle By Name(w451) -> ("Channel Table"=w454:T8, "ModelList Num"=w452:i32, "Model List name"=w453:string[])
            n167 = Delete From Array(array=w454, length=1, index=w452) -> (array with subset deleted=w449:T8)  [unwired: 1 out]
            n168 = Delete From Array(array=w453, length=1, index=w452) -> (array with subset deleted=w448:string[])  [unwired: 1 out]
            n169 = Bundle By Name(cluster=w451, "Channel Table"=w449, "Model List name"=w448) -> (w450:T10)
            n170 = Enqueue Element At Opposite End(queue=w460, element=cluster{"State":T12, "Data":variant} {"State"=enum."Update", "Data"=variant}, error in (no error)=w457) -> (queue out=w459:refnum<queue>, error out=w458:errorcluster)  [unwired: 1 in, 1 out]
          }
          frame "Set Time" {
            n171 = Variant To Data(error in=w469, type=0, Variant=w468) -> (data=w463:i32, error out=w462:errorcluster)
            n172 = Bundle By Name(cluster=w465, "Set Time"=w463) -> (w464:T10)
          }
          frame "Test" {
            n173 = Unbundle By Name(w479) -> ("Channel 1 Wave"=w478:waveform(dbl), "Channel 2 Wave"=w477:waveform(dbl), "Channel 3 Wave"=w476:waveform(dbl), "Channel 4 Wave"=w475:waveform(dbl))
            n174 = Build Array(w478, w477, w476, w475) -> (w473:waveform(dbl)[])
            n175 = property on="Test Setting" class="Arr (strict)"("Value"=w473) -> (error out=w470:errorcluster)  [unwired: 2 in, 1 out]
            n176 = property on="Test State" class="Enum (strict)"(error in=w470, "Value"=Test_State."Normal" ("Test State")) -> (error out=w471:errorcluster)  [unwired: 1 in, 1 out]
            n177 = Enqueue Element(queue=w482, element=cluster{"State":T12, "Data":variant} {"State"=enum."Start Time", "Data"=variant}, error in (no error)=w484) -> (queue out=w481:refnum<queue>, error out=w483:errorcluster)  [unwired: 1 in, 1 out]
            n178 = property on="Testing?" class="Bool (strict)"(error in=w471, "Value"=TRUE ("Testing?")) -> ()  [unwired: 1 in, 2 out]
            n179 = Bundle By Name(cluster=w479, "Button"=FALSE, "Testing"=TRUE) -> (w487:T10)
          }
          frame "Start Time" {
            n180 = Unbundle By Name(w492) -> ("Button Time"=w490:i32, "Button"=w491:bool, "Set Time"=w489:i32)
            n181 = Select(t=w490, s=w491, f=w489) -> (s? t:f=w488:i32)
            n182 = call "FGV_Timer.vi"("State"=Timer_State."Start", "error in (no error)"=w500, "Set Time"=w488) -> ("error out"=w494:errorcluster)  [unwired: 6 in, 2 out]
            n183 = Bundle By Name(cluster=w492, "Elapse Time"=0.0) -> (w496:T10)
            n184 = Enqueue Element(queue=w499, element=cluster{"State":T12, "Data":variant} {"State"=enum."Check Time", "Data"=variant}, error in (no error)=w494) -> (queue out=w498:refnum<queue>, error out=w497:errorcluster)  [unwired: 1 in, 1 out]
          }
          frame "Check Time" {
            n185 = call "FGV_Timer.vi"("State"=Timer_State."Check", "error in (no error)"=w511) -> ("error out"=w505:errorcluster, "Elapsed Time"=w503:dbl, "Elapsed ?"=w502:bool)  [unwired: 7 in]
            n186 = case shown="True" w502 {
              frame False {
              }
              frame True {
                n187 = property on="Testing?" class="Bool (strict)"("Value"=FALSE ("Testing?")) -> ()  [unwired: 2 in, 2 out]
              }
            }
            n188 = Bundle By Name(cluster=w507, "Elapsed ?"=w502, "Elapse Time"=w503) -> (w506:T10)
            n189 = Enqueue Element(queue=w510, element=cluster{"State":T12, "Data":variant} {"State"=enum."Update", "Data"=variant}, error in (no error)=w505) -> (queue out=w509:refnum<queue>, error out=w508:errorcluster)  [unwired: 1 in, 1 out]
          }
          frame "Save" {
            n190 = Unbundle By Name(w522) -> ("Project Path"=w517:path, "Project List name"=w518:string[], "ProjectList Num"=w519:i32, "Channel Table"=w524:T8, "Model List name"=w523:string[])
            n191 = Index Array(array=w518, index=w519) -> (element=w516:string)
            n192 = Build Path(base path=w517, name or relative path=w516) -> (appended path=w515:path)
            n193 = Bundle("Channel Table"=w524, "Model List name"=w523) -> (w526:T24)  [unwired: 1 in]
            n194 = Flatten To XML(anything=w526) -> (xml string=w525:string)
            n195 = Build Path(base path=w515, name or relative path="Channel Setting.dat") -> (appended path=w527:path)
            n196 = call-poly <vilib>:"Write to XML File.vi"("XML Input"=w525, "XML File Path"=w527) -> ()  [unwired: 7 in, 3 out]
          }
          frame "Frontward" {
            n197 = Unbundle("Front") -> ("Channel 1"=w541:T25, "Channel 2"=w542:T26, "Channel 3"=w543:T27, "Channel 4"=w544:T26)
            n198 = Build Array(w541, w542, w543, w544) -> (w540:T28)
            n199 = for {
              tunnel: w540 -> [w553] mode=indexing
              tunnel: [w554] -> w539 mode=indexing
              n200 = Unbundle By Name(w553) -> ("offset"=w555:dbl, "signal type 1"=w556:T19, "frequency 1"=w557:i32, "amplitude 1"=w558:dbl, "phase"=w559:dbl)
              n201 = call <vilib>:"Basic Function Generator.vi"("offset"=w555, "reset signal"=TRUE, "sampling info"=cluster{"Fs":dbl, "#s":dbl} {"Fs"=1000.0, "#s"=100.0} ("sampling info 4"), "signal type"=w556, "phase"=w559, "amplitude"=w558, "frequency"=w557) -> ("signal out"=w554:waveform(dbl))  [unwired: 2 in, 2 out]
            }
            n202 = property on="Test Setting" class="Arr (strict)"("Value"=w539) -> (error out=w537:errorcluster)  [unwired: 2 in, 1 out]
            n203 = Index Array(array=w539) -> (element #1=→"Channel 1 Wave (Main)":waveform(dbl), element #2=→"Channel 2 Wave (Main)":waveform(dbl), element #3=→"Channel 3 Wave (Main)":waveform(dbl), element #4=→"Channel 4 Wave (Main)":waveform(dbl))  [unwired: 4 in]
            n204 = property on="Test State" class="Enum (strict)"(error in=w537, "Value"=Test_State."Normal" ("Test State")) -> (error out=w536:errorcluster)  [unwired: 1 in, 1 out]
            n205 = Enqueue Element At Opposite End(queue=w552, element=cluster{"State":T12, "Data":variant} {"State"=enum."Start Time", "Data"=variant}, error in (no error)=w549) -> (queue out=w551:refnum<queue>, error out=w548:errorcluster)  [unwired: 1 in, 1 out]
            n206 = property on="Testing?" class="Bool (strict)"(error in=w536, "Value"=TRUE ("Testing?")) -> ()  [unwired: 1 in, 2 out]
            n207 = Bundle By Name(cluster=w547, "Button"=TRUE, "Button Time"=60000 ("Set Time"), "Testing"=TRUE) -> (w546:T10)
          }
          frame "Leftward" {
            w566 = TRUE ("Testing")
            n208 = Unbundle("Left") -> ("Channel 1"=w574:T29, "Channel 2"=w575:T30, "Channel 3"=w576:T30, "Channel 4"=w577:T31)
            n209 = Build Array(w574, w575, w576, w577) -> (w573:T32)
            n210 = for {
              tunnel: w573 -> [w586] mode=indexing
              tunnel: [w587] -> w571 mode=indexing
              n211 = Unbundle By Name(w586) -> ("offset"=w588:i32, "signal type 1"=w589:T19, "frequency 1"=w590:i32, "amplitude 1"=w591:dbl, "phase"=w592:dbl)
              n212 = call <vilib>:"Basic Function Generator.vi"("offset"=w588, "reset signal"=TRUE, "sampling info"=cluster{"Fs":dbl, "#s":dbl} {"Fs"=1000.0, "#s"=100.0} ("sampling info 4"), "signal type"=w589, "phase"=w592, "amplitude"=w591, "frequency"=w590) -> ("signal out"=w587:waveform(dbl))  [unwired: 2 in, 2 out]
            }
            n213 = Index Array(array=w571) -> (element #1=w565:waveform(dbl), element #2=w564:waveform(dbl), element #3=w563:waveform(dbl), element #4=w562:waveform(dbl))  [unwired: 4 in]
            n214 = property on="Test Setting" class="Arr (strict)"("Value"=w571) -> (error out=w570:errorcluster)  [unwired: 2 in, 1 out]
            n215 = property on="Channel 1 Wave (Main)" class="WFGraph (strict)"("Value"=w565) -> ()  [unwired: 2 in, 2 out]
            n216 = property on="Channel 2 Wave (Main)" class="WFGraph (strict)"("Value"=w564) -> ()  [unwired: 2 in, 2 out]
            n217 = property on="Channel 3 Wave (Main)" class="WFGraph (strict)"("Value"=w563) -> ()  [unwired: 2 in, 2 out]
            n218 = property on="Channel 4 Wave (Main)" class="WFGraph (strict)"("Value"=w562) -> ()  [unwired: 2 in, 2 out]
            n219 = property on="Test State" class="Enum (strict)"(error in=w570, "Value"=Test_State."Normal" ("Test State")) -> (error out=w569:errorcluster)  [unwired: 1 in, 1 out]
            n220 = Enqueue Element At Opposite End(queue=w585, element=cluster{"State":T12, "Data":variant} {"State"=enum."Start Time", "Data"=variant}, error in (no error)=w582) -> (queue out=w584:refnum<queue>, error out=w581:errorcluster)  [unwired: 1 in, 1 out]
            n221 = property on="Testing?" class="Bool (strict)"(error in=w569, "Value"=TRUE ("Testing?")) -> ()  [unwired: 1 in, 2 out]
            n222 = Bundle By Name(cluster=w580, "Button Time"=60000 ("Set Time"), "Button"=w566, "Testing"=w566) -> (w579:T10)
          }
          frame "Backward" {
            w599 = TRUE ("Testing")
            n223 = Unbundle("Back") -> ("Channel 1"=w607:T27, "Channel 2"=w608:T25, "Channel 3"=w609:T30, "Channel 4"=w610:T26)
            n224 = Build Array(w607, w608, w609, w610) -> (w606:T28)
            n225 = for {
              tunnel: w606 -> [w619] mode=indexing
              tunnel: [w620] -> w604 mode=indexing
              n226 = Unbundle By Name(w619) -> ("offset"=w621:dbl, "signal type 1"=w622:T19, "frequency 1"=w623:i32, "amplitude 1"=w624:dbl, "phase"=w625:dbl)
              n227 = call <vilib>:"Basic Function Generator.vi"("offset"=w621, "reset signal"=TRUE, "sampling info"=cluster{"Fs":dbl, "#s":dbl} {"Fs"=1000.0, "#s"=100.0} ("sampling info 4"), "signal type"=w622, "phase"=w625, "amplitude"=w624, "frequency"=w623) -> ("signal out"=w620:waveform(dbl))  [unwired: 2 in, 2 out]
            }
            n228 = Index Array(array=w604) -> (element #1=w598:waveform(dbl), element #2=w597:waveform(dbl), element #3=w596:waveform(dbl), element #4=w595:waveform(dbl))  [unwired: 4 in]
            n229 = property on="Test Setting" class="Arr (strict)"("Value"=w604) -> (error out=w601:errorcluster)  [unwired: 2 in, 1 out]
            n230 = property on="Channel 1 Wave (Main)" class="WFGraph (strict)"("Value"=w598) -> ()  [unwired: 2 in, 2 out]
            n231 = property on="Channel 2 Wave (Main)" class="WFGraph (strict)"("Value"=w597) -> ()  [unwired: 2 in, 2 out]
            n232 = property on="Channel 3 Wave (Main)" class="WFGraph (strict)"("Value"=w596) -> ()  [unwired: 2 in, 2 out]
            n233 = property on="Channel 4 Wave (Main)" class="WFGraph (strict)"("Value"=w595) -> ()  [unwired: 2 in, 2 out]
            n234 = property on="Test State" class="Enum (strict)"(error in=w601, "Value"=Test_State."Normal" ("Test State")) -> (error out=w602:errorcluster)  [unwired: 1 in, 1 out]
            n235 = Enqueue Element At Opposite End(queue=w618, element=cluster{"State":T12, "Data":variant} {"State"=enum."Start Time", "Data"=variant}, error in (no error)=w615) -> (queue out=w617:refnum<queue>, error out=w614:errorcluster)  [unwired: 1 in, 1 out]
            n236 = property on="Testing?" class="Bool (strict)"(error in=w602, "Value"=TRUE ("Testing?")) -> ()  [unwired: 1 in, 2 out]
            n237 = Bundle By Name(cluster=w613, "Button Time"=60000 ("Set Time"), "Testing"=w599, "Button"=w599) -> (w612:T10)
          }
          frame "Rightward" {
            w632 = TRUE ("Testing")
            n238 = Unbundle("Right") -> ("Channel 1"=w640:T25, "Channel 2"=w641:T27, "Channel 3"=w642:T26, "Channel 4"=w643:T26)
            n239 = Build Array(w640, w641, w642, w643) -> (w639:T28)
            n240 = for {
              tunnel: w639 -> [w652] mode=indexing
              tunnel: [w653] -> w638 mode=indexing
              n241 = Unbundle By Name(w652) -> ("offset"=w654:dbl, "signal type 1"=w655:T19, "frequency 1"=w656:i32, "amplitude 1"=w657:dbl, "phase"=w658:dbl)
              n242 = call <vilib>:"Basic Function Generator.vi"("offset"=w654, "reset signal"=TRUE, "sampling info"=cluster{"Fs":dbl, "#s":dbl} {"Fs"=1000.0, "#s"=100.0} ("sampling info 4"), "signal type"=w655, "phase"=w658, "amplitude"=w657, "frequency"=w656) -> ("signal out"=w653:waveform(dbl))  [unwired: 2 in, 2 out]
            }
            n243 = property on="Test Setting" class="Arr (strict)"("Value"=w638) -> (error out=w635:errorcluster)  [unwired: 2 in, 1 out]
            n244 = Index Array(array=w638) -> (element #1=w631:waveform(dbl), element #2=w630:waveform(dbl), element #3=w629:waveform(dbl), element #4=w628:waveform(dbl))  [unwired: 4 in]
            n245 = property on="Channel 1 Wave (Main)" class="WFGraph (strict)"("Value"=w631) -> ()  [unwired: 2 in, 2 out]
            n246 = property on="Channel 2 Wave (Main)" class="WFGraph (strict)"("Value"=w630) -> ()  [unwired: 2 in, 2 out]
            n247 = property on="Channel 3 Wave (Main)" class="WFGraph (strict)"("Value"=w629) -> ()  [unwired: 2 in, 2 out]
            n248 = property on="Channel 4 Wave (Main)" class="WFGraph (strict)"("Value"=w628) -> ()  [unwired: 2 in, 2 out]
            n249 = property on="Test State" class="Enum (strict)"(error in=w635, "Value"=Test_State."Normal" ("Test State")) -> (error out=w634:errorcluster)  [unwired: 1 in, 1 out]
            n250 = Enqueue Element At Opposite End(queue=w651, element=cluster{"State":T12, "Data":variant} {"State"=enum."Start Time", "Data"=variant}, error in (no error)=w648) -> (queue out=w650:refnum<queue>, error out=w647:errorcluster)  [unwired: 1 in, 1 out]
            n251 = property on="Testing?" class="Bool (strict)"(error in=w634, "Value"=TRUE ("Testing?")) -> ()  [unwired: 1 in, 2 out]
            n252 = Bundle By Name(cluster=w646, "Button Time"=60000 ("Set Time"), "Button"=w632, "Testing"=w632) -> (w645:T10)
          }
          frame "Stop" {
            n253 = property on="Testing?" class="Bool (strict)"("Value"=FALSE ("Testing?")) -> ()  [unwired: 2 in, 2 out]
            n254 = Enqueue Element At Opposite End(queue=w669, element=cluster{"State":T12, "Data":variant} {"State"=enum."Idle", "Data"=variant}, error in (no error)=w667) -> (queue out=w668:refnum<queue>, error out=w666:errorcluster)  [unwired: 1 in, 1 out]
            n255 = Bundle By Name(cluster=w664, "Stop"=TRUE) -> (w663:T10)
          }
          frame "Center" {
            w670 = TRUE ("Center/Bump")
            n256 = property on="Test State" class="Enum (strict)"("Value"=Test_State."Center" ("Test State")) -> (error out=w672:errorcluster)  [unwired: 2 in, 1 out]
            n257 = property on="Testing?" class="Bool (strict)"(error in=w672, "Value"=TRUE ("Testing?")) -> ()  [unwired: 1 in, 2 out]
            n258 = Enqueue Element(queue=w680, element=cluster{"State":T12, "Data":variant} {"State"=enum."Start Time", "Data"=variant}, error in (no error)=w679) -> (queue out=w677:refnum<queue>, error out=w678:errorcluster)  [unwired: 1 in, 1 out]
            n259 = Bundle By Name(cluster=w676, "Button Time"=60000, "Button"=w670, "Testing"=w670) -> (w675:T10)
          }
          frame "Bump" {
            w682 = TRUE ("Center/Bump")
            n260 = property on="Test State" class="Enum (strict)"("Value"=Test_State."Bump" ("Test State")) -> (error out=w684:errorcluster)  [unwired: 2 in, 1 out]
            n261 = property on="Testing?" class="Bool (strict)"(error in=w684, "Value"=TRUE ("Testing?")) -> ()  [unwired: 1 in, 2 out]
            n262 = Enqueue Element(queue=w692, element=cluster{"State":T12, "Data":variant} {"State"=enum."Start Time", "Data"=variant}, error in (no error)=w691) -> (queue out=w689:refnum<queue>, error out=w690:errorcluster)  [unwired: 1 in, 1 out]
            n263 = Bundle By Name(cluster=w688, "Button Time"=60000, "Button"=w682, "Testing"=w682) -> (w687:T10)
          }
          frame "Add Project" {
            n264 = Unbundle By Name(w699) -> ("Project Path"=w700:path, "Project List name"=w697:string[], "Project Name(Set)"=w694:string)
            n265 = Search 1D Array(1D array=w697, element=w694) -> (index of element=w696:i32)  [unwired: 1 in]
            n266 = Greater Or Equal To 0?(x=w696) -> (x >= 0?=w695:bool)
            n267 = case shown="False" w695 {
              tunnel: w700 -> [w719 w730]
              tunnel: w699 -> [w714 w721]
              tunnel: [w718 w721] -> w698
              tunnel: w694 -> [w716 w729]
              frame False {
                n268 = Unbundle By Name(w714) -> ("Channel Table"=w713:T8, "Model List name"=w712:string[])
                n269 = Build Path(base path=w719, name or relative path=w716) -> (appended path=w708:path)
                n270 = Create Folder(path (use dialog)=w708) -> (error out=w720:errorcluster)  [unwired: 2 in, 2 out]
                n271 = Bundle("Channel Table"=w713, "Model List name"=w712) -> (w711:T24)  [unwired: 1 in]
                n272 = List Folder(path=w719, error in=w720) -> (folder names=w717:string[], error out=w706:errorcluster)  [unwired: 2 in, 2 out]
                n273 = Flatten To XML(anything=w711) -> (xml string=w715:string)
                n274 = Build Path(base path=w708, name or relative path="Channel Setting.dat") -> (appended path=w709:path)
                n275 = call-poly <vilib>:"Write to XML File.vi"("error in (no error)"=w706, "XML Input"=w715, "XML File Path"=w709) -> ()  [unwired: 6 in, 3 out]
                n276 = Bundle By Name(cluster=w714, "Project List name"=w717, "Project Name(Set)"="") -> (w718:T10)
              }
              frame True {
                n277 = Unbundle By Name(w721) -> ("Channel Table"=w727:T8, "Model List name"=w726:string[])
                n278 = Build Path(base path=w730, name or relative path=w729) -> (appended path=w722:path)
                n279 = Bundle("Channel Table"=w727, "Model List name"=w726) -> (w725:T24)  [unwired: 1 in]
                n280 = Flatten To XML(anything=w725) -> (xml string=w728:string)
                n281 = Build Path(base path=w722, name or relative path="Channel Setting.dat") -> (appended path=w723:path)
                n282 = call-poly <vilib>:"Write to XML File.vi"("XML Input"=w728, "XML File Path"=w723) -> ()  [unwired: 7 in, 3 out]
              }
            }
            n283 = Enqueue Element At Opposite End(queue=w705, element=cluster{"State":T12, "Data":variant} {"State"=enum."Update", "Data"=variant}, error in (no error)=w702) -> (queue out=w704:refnum<queue>, error out=w701:errorcluster)  [unwired: 1 in, 1 out]
          }
          frame "Remove Project" {
            n284 = Unbundle By Name(w739) -> ("Project Path"=w733:path, "Project List name"=w737:string[], "ProjectList Num"=w736:i32)
            n285 = Index Array(array=w737, index=w736) -> (element=w735:string)
            n286 = Build Path(base path=w733, name or relative path=w735) -> (appended path=w734:path)
            n287 = Delete(path (use dialog)=w734) -> (error out=w732:errorcluster)  [unwired: 4 in, 2 out]
            n288 = List Folder(path=w733, error in=w732) -> (folder names=w731:string[])  [unwired: 2 in, 3 out]
            n289 = Bundle By Name(cluster=w739, "Project List name"=w731) -> (w738:T10)
            n290 = Enqueue Element At Opposite End(queue=w744, element=cluster{"State":T12, "Data":variant} {"State"=enum."Update", "Data"=variant}, error in (no error)=w741) -> (queue out=w743:refnum<queue>, error out=w740:errorcluster)  [unwired: 1 in, 1 out]
          }
          frame "Project List" {
            n291 = Variant To Data(error in=w747, type=0 ("NewVal"), Variant=w748) -> (data=w745:i32, error out=w746:errorcluster)
            n292 = Bundle By Name(cluster=w751, "ProjectList Num"=w745) -> (w750:T10)
            n293 = Enqueue Element At Opposite End(queue=w755, element=cluster{"State":T12, "Data":variant} {"State"=enum."Update", "Data"=variant}, error in (no error)=w746) -> (queue out=w754:refnum<queue>, error out=w752:errorcluster)  [unwired: 1 in, 1 out]
          }
          frame "Project Name" {
            n294 = Variant To Data(error in=w758, type="" ("NewVal"), Variant=w759) -> (data=w756:string, error out=w757:errorcluster)
            n295 = Bundle By Name(cluster=w762, "Project Name(Set)"=w756) -> (w761:T10)
            n296 = Enqueue Element At Opposite End(queue=w766, element=cluster{"State":T12, "Data":variant} {"State"=enum."Update", "Data"=variant}, error in (no error)=w757) -> (queue out=w765:refnum<queue>, error out=w763:errorcluster)  [unwired: 1 in, 1 out]
          }
          frame "Project OK" {
            n297 = Unbundle By Name(w773) -> ("Project Path"=w772:path, "Project List name"=w768:string[], "ProjectList Num"=w769:i32)
            n298 = Empty Array?(array=w768) -> (empty?=w767:bool)
            n299 = case shown="False" w767 {
              tunnel: [w795 w806] -> w774
              tunnel: w773 -> [w788 w806]
              tunnel: w772 -> [w787 _]
              tunnel: w771 -> [w786 w807]
              tunnel: [w785 w807] -> w770
              tunnel: w768 -> [w784 _]
              tunnel: w769 -> [w783 _]
              frame False {
                n300 = Index Array(array=w784, index=w783) -> (element=w779:string)
                n301 = Build Path(base path=w787, name or relative path=w779) -> (appended path=w789:path)
                n302 = Build Path(base path=w789, name or relative path="Channel Setting.dat") -> (appended path=w792:path)
                n303 = call <vilib>:"Check if File or Folder Exists.vi"("error in (no error)"=w786, "path"=w792) -> ("error out"=w793:errorcluster, "file or folder exists?"=w791:bool, "dup path"=w790:path)  [unwired: 7 in]
                n304 = case shown="True" w791 {
                  tunnel: [w796 w800] -> w785
                  tunnel: w793 -> [w796 w799]
                  tunnel: w790 -> [_ w798]
                  tunnel: [_ w797] -> w782
                  frame False {
                  }
                  frame True {
                    n305 = call-poly <vilib>:"Read From XML File.vi"("error in (no error)"=w799, "XML File Path"=w798) -> ("error out"=w801:errorcluster, "XML Elements"=w805:string)  [unwired: 7 in, 1 out]
                    n306 = Bundle("DataTable"=T8 [], "Item Names"=string[] []) -> (w802:T18)  [unwired: 1 in]
                    n307 = Unflatten From XML(xml string=w805, type=w802, error in (no error)=w801) -> (value=w797:T18, error out=w800:errorcluster)
                  }
                }
                n308 = Unbundle(w782) -> ("DataTable"=w781:T8, "Item Names"=w780:string[])
                n309 = Bundle By Name(cluster=w788, "Channel Table"=w781, "Model List name"=w780, "Project Name"=w779) -> (w795:T10)
              }
              frame True {
              }
            }
            n310 = Enqueue Element At Opposite End(queue=w778, element=cluster{"State":T12, "Data":variant} {"State"=enum."Update", "Data"=variant}, error in (no error)=w770) -> (queue out=w777:refnum<queue>, error out=w775:errorcluster)  [unwired: 1 in, 1 out]
          }
          frame "Exit" {
            w809 = TRUE
            n311 = call "FGV_EXIT.vi"("Function"=enum16{"Read", "Write"}."Write", "EXIT"=w809) -> ()  [unwired: 6 in, 1 out]
          }
        }
        n312 = call "FGV_EXIT.vi"("Function"=enum16{"Read", "Write"}."Read") -> ("EXIT out"=w177:bool)  [unwired: 7 in]
        n313 = Or(x=w175, y=w177) -> (x .or. y?=w176:bool)
        n314 = case shown="True" w176 {
          tunnel: w186 -> [w195 w204]
          tunnel: w185 -> [w196 w205]
          tunnel: [w196 w205] -> w184
          tunnel: [w195 w201] -> w183
          tunnel: [w194 w200] -> w182
          tunnel: w175 -> [w194 w198]
          frame False {
          }
          frame True {
            n315 = call <vilib>:"Clear Errors.vi"("error in (no error)"=w198) -> ("error out"=w197:errorcluster)  [unwired: 5 in, 1 out]
            n316 = Flush Queue(queue=w204, error in (no error)=w197) -> (queue out=w202:refnum<queue>, error out=w203:errorcluster)  [unwired: 1 out]
            n317 = Enqueue Element(queue=w202, element=cluster{"State":T12, "Data":variant} {"State"=enum."Exit", "Data"=variant}, error in (no error)=w203) -> (queue out=w201:refnum<queue>, error out=w200:errorcluster)  [unwired: 1 in, 1 out]
          }
        }
      }
      n318 = while {
        tunnel: w29 -> [w40]
        tunnel: w27 -> [w33]
        tunnel: w25 -> [w31]
        stop <- w38 stop-if-true
        n319 = call <vilib>:"TCP Listen.vi"("error in (no error)"=w33, "timeout ms (wait forever: -1)"=1000, "port"=u16 6025) -> ("error out"=w36:errorcluster, "connection ID"=w35:refnum<k5>)  [unwired: 4 in, 3 out]
        n320 = Wait (ms)(milliseconds to wait=u32 1) -> ()  [unwired: 1 out]
        n321 = case shown="No Error" w36 {
          selector: w36 -> [w49 w126]
          tunnel: [w43 w124] -> _
          tunnel: w35 -> [w50 _]
          tunnel: w40 -> [w48 _]
          tunnel: w31 -> [w45 _]
          frame No Error {
            n322 = while {
              tunnel: w49 -> [w117]
              tunnel: w50 -> [w116]
              tunnel: w48 -> [w115]
              tunnel: [w109] -> w47
              stop <- w108 stop-if-true
              n323 = Dequeue Element(queue=w115, timeout in ms (-1)=100, error in (no error)=w117) -> (element=w105:string, error out=w118:errorcluster)  [unwired: 2 out]
              n324 = To Lower Case(string=w105) -> (all lower case string=w104:string)
              n325 = Empty String/Path?(string/path=w105) -> (empty?=w110:bool)
              n326 = Equal?(x=w104, y="close") -> (x = y?=w107:bool)
              n327 = case shown="False" w110 {
                tunnel: w105 -> [w122 _]
                tunnel: w118 -> [w121 w123]
                tunnel: w116 -> [w120 _]
                tunnel: [w119 w123] -> w109
                frame False {
                  n328 = TCP Write(connection ID=w120, data in=w122, error in (no error)=w121) -> (error out=w119:errorcluster)  [unwired: 1 in, 2 out]
                }
                frame True {
                }
              }
              n329 = call "FGV_EXIT.vi"("Function"=enum16{"Read", "Write"}."Read") -> ("EXIT out"=w111:bool)  [unwired: 7 in]
              n330 = property on="TCP connect" class="Bool (strict)"() -> ("Value"=w103:bool)  [unwired: 2 in, 2 out]
              n331 = Wait (ms)(milliseconds to wait=u32 1) -> ()  [unwired: 1 out]
              n332 = Compound Arithmetic op=OR(w109, w103, w107, w111) -> (w108:bool)
            }
            n333 = while {
              tunnel: w50 -> [w68]
              tunnel: w49 -> [w67]
              tunnel: [w59] -> w46
              tunnel: w45 -> [w55]
              stop <- w54 stop-if-true
              w64 = 56 items=["No Error", "Argument Error", "Memory Full", "Out of Zone", "End of File", "File Already Open", "Generic File IO Error", "File Not Found", "File Permission Error", "Disk Full", "Duplicate Path", "Too Many Files Open", "Not Enabled", "Resource File Not Found", "Cannot Add Resource", "Resource Not Found", "Image Not Found", "Image Memory Error", "Pen Does Not Exist", "Config Bad Type", "Config Token Not Found", "Config Parse Error", "Config Memory Error", "Bad External Code Format", "Bad External Code Offset", "External Code Not Present", "Null Window", "Destroy Window Mixup", "Null Menu", "Print Aborted", "Bad Print Record", "Print Driver Error", "Windows Error During Print", "Memory Error During Print", "Print Dialog Error", "Generic Print Error", "Invalid Device Refnum", "Device Not Found", "Device Parameter Error", "Device Unit Error", "Can't Open Device", "Device Call Aborted", "Generic Error", "Cancelled By User", "Object ID Too Low", "Object ID Too High", "Object Not In Heap", "Unknown Heap", "Bad DefProc ID", "DefProc Not In Table", "Message Out Of Range", "Null Method", "Unknown Message", "Manager Call Not Supported", "Bad address", "Connection In progress", "Connection timed out", "Connection is already in progress", "Network attribute not supported", "Network error", "Address in use", "System out of memory", "Connection aborted", "Connection refused", "Connection is not connected", "Connection is already connected", "Connection closed", "Initialize error (interapplication manager)", "Bad occurrence", "Wait on unbound occurrence handler", "Occurrence queue overflow", "Bad path", "Semaphore not signaled", "Unrecognized type (interapplication manager)"] ("1st Error to Convert")
              n334 = TCP Read(connection ID=w68, bytes to read=5000, error in (no error)=w67, 7:T11."Standard" ("mode (standard)"), 9:100 ("timeout ms (25000)")) -> (data out=w66:string, error out=w65:errorcluster)  [unwired: 1 out]
              n335 = Wait (ms)(milliseconds to wait=u32 1) -> ()  [unwired: 1 out]
              n336 = call <vilib>:"Trim Whitespace.vi"("string"=w66) -> ("trimmed string"=w57:string)  [unwired: 1 in]
              n337 = call <vilib>:"Error to Warning.vi"("1st Error to Convert"=w64, "error in"=w65) -> ("warning out"=w52:errorcluster)  [unwired: 13 in]
              n338 = Empty String/Path?(string/path=w57) -> (empty?=w63:bool)
              n339 = To Lower Case(string=w57) -> (all lower case string=w56:string)
              n340 = case shown="False" w63 {
                tunnel: w52 -> [w73 w102]
                tunnel: [w72 w102] -> w59
                tunnel: w56 -> [w71 _]
                tunnel: w55 -> [w70 _]
                frame False {
                  n341 = case shown="\"stop\", Default" w71 {
                    tunnel: w73 -> [w76 w81 w85 w88 w93 w97 w100]
                    tunnel: [w75 w79 w84 w87 w92 w96 w99] -> w72
                    tunnel: w70 -> [w74 w80 w83 w86 w91 w94 w98]
                    frame "stop", Default {
                      n342 = Enqueue Element(queue=w74, element=cluster{"State":T12, "Data":variant} {"State"=enum."Stop", "Data"=variant}, error in (no error)=w76) -> (error out=w75:errorcluster)  [unwired: 1 in, 2 out]
                    }
                    frame "front" {
                      n343 = Enqueue Element(queue=w80, element=cluster{"State":T12, "Data":variant} {"State"=enum."Frontward", "Data"=variant}, error in (no error)=w81) -> (error out=w79:errorcluster)  [unwired: 1 in, 2 out]
                    }
                    frame "bump" {
                      n344 = Enqueue Element(queue=w83, element=cluster{"State":T12, "Data":variant} {"State"=enum."Bump", "Data"=variant}, error in (no error)=w85) -> (error out=w84:errorcluster)  [unwired: 1 in, 2 out]
                    }
                    frame "center" {
                      n345 = Enqueue Element(queue=w86, element=cluster{"State":T12, "Data":variant} {"State"=enum."Center", "Data"=variant}, error in (no error)=w88) -> (error out=w87:errorcluster)  [unwired: 1 in, 2 out]
                    }
                    frame "right" {
                      n346 = Enqueue Element(queue=w91, element=cluster{"State":T12, "Data":variant} {"State"=enum."Rightward", "Data"=variant}, error in (no error)=w93) -> (error out=w92:errorcluster)  [unwired: 1 in, 2 out]
                    }
                    frame "back" {
                      n347 = Enqueue Element(queue=w94, element=cluster{"State":T12, "Data":variant} {"State"=enum."Backward", "Data"=variant}, error in (no error)=w97) -> (error out=w96:errorcluster)  [unwired: 1 in, 2 out]
                    }
                    frame "left" {
                      n348 = Enqueue Element(queue=w98, element=cluster{"State":T12, "Data":variant} {"State"=enum."Leftward", "Data"=variant}, error in (no error)=w100) -> (error out=w99:errorcluster)  [unwired: 1 in, 2 out]
                    }
                  }
                }
                frame True {
                  # "Wait CMD"
                }
              }
              n349 = Unbundle By Name(w52) -> ("status"=→"TCP connect":bool)
              n350 = call "FGV_EXIT.vi"("Function"=enum16{"Read", "Write"}."Read") -> ("EXIT out"=w53:bool)  [unwired: 7 in]
              n351 = Or(x=w53, y=w52) -> (x .or. y?=w54:bool)
            }
            n352 = Merge Errors(w47, w46) -> (w44:errorcluster)
            n353 = call <vilib>:"Clear Errors.vi"("error in (no error)"=w44) -> ("error out"=w41:errorcluster)  [unwired: 5 in, 1 out]
            n354 = property on="TCP connect" class="Bool (strict)"(error in=w41, "Value"=FALSE ("TCP connect")) -> (error out=w43:errorcluster)  [unwired: 1 in, 1 out]
          }
          frame Error {
            w125 = 56 items=["No Error", "Argument Error", "Memory Full", "Out of Zone", "End of File", "File Already Open", "Generic File IO Error", "File Not Found", "File Permission Error", "Disk Full", "Duplicate Path", "Too Many Files Open", "Not Enabled", "Resource File Not Found", "Cannot Add Resource", "Resource Not Found", "Image Not Found", "Image Memory Error", "Pen Does Not Exist", "Config Bad Type", "Config Token Not Found", "Config Parse Error", "Config Memory Error", "Bad External Code Format", "Bad External Code Offset", "External Code Not Present", "Null Window", "Destroy Window Mixup", "Null Menu", "Print Aborted", "Bad Print Record", "Print Driver Error", "Windows Error During Print", "Memory Error During Print", "Print Dialog Error", "Generic Print Error", "Invalid Device Refnum", "Device Not Found", "Device Parameter Error", "Device Unit Error", "Can't Open Device", "Device Call Aborted", "Generic Error", "Cancelled By User", "Object ID Too Low", "Object ID Too High", "Object Not In Heap", "Unknown Heap", "Bad DefProc ID", "DefProc Not In Table", "Message Out Of Range", "Null Method", "Unknown Message", "Manager Call Not Supported", "Bad address", "Connection In progress", "Connection timed out", "Connection is already in progress", "Network attribute not supported", "Network error", "Address in use", "System out of memory", "Connection aborted", "Connection refused", "Connection is not connected", "Connection is already connected", "Connection closed", "Initialize error (interapplication manager)", "Bad occurrence", "Wait on unbound occurrence handler", "Occurrence queue overflow", "Bad path", "Semaphore not signaled", "Unrecognized type (interapplication manager)"] ("1st Error to Convert")
            n355 = call <vilib>:"Error to Warning.vi"("1st Error to Convert"=w125, "error in"=w126) -> ("warning out"=w124:errorcluster)  [unwired: 13 in]
          }
        }
        n356 = call "FGV_EXIT.vi"("Function"=enum16{"Read", "Write"}."Read") -> ("EXIT out"=w38:bool)  [unwired: 7 in]
      }
      n357 = while {
        stop <- w129 stop-if-true
        n358 = property on="Testing?" class="Bool (strict)"() -> ("Value"=w128:bool)  [unwired: 2 in, 2 out]
        n359 = Wait (ms)(milliseconds to wait=u32 1) -> ()  [unwired: 1 out]
        n360 = case shown="True" w128 {
          frame False {
          }
          frame True {
            n361 = property on="Test State" class="Enum (strict)"() -> ("Value"=w131:T7)  [unwired: 2 in, 2 out]
            n362 = case shown="\"Bump\"" w131 {
              frame "Normal", Default {
                n363 = property on="Test Setting" class="Arr (strict)"() -> ("Value"=w132:waveform(dbl)[])  [unwired: 2 in, 2 out]
                n364 = call "DAQ Assistant"("data"=w132) -> ()  [unwired: 17 in, 2 out]
                n365 = disable-structure shown="Disabled" {
                  frame Disabled {
                    # "daq2"
                    n366 = call "DAQ Assistant2"() -> ()  [unwired: 18 in, 2 out]
                  }
                  frame Enabled {
                  }
                }
              }
              frame "Bump" {
                n367 = Unbundle("Bump") -> ("Channel 1"=w143:T29, "Channel 2"=w142:T29, "Channel 3"=w141:T29, "Channel 4"=w140:T29)
                n368 = Build Array(w143, w142, w141, w140) -> (w139:T32)
                n369 = for {
                  tunnel: w139 -> [w146] mode=indexing
                  tunnel: [w147] -> w134 mode=indexing
                  n370 = Unbundle By Name(w146) -> ("offset"=w148:i32, "signal type 1"=w149:T19, "frequency 1"=w150:i32, "amplitude 1"=w151:dbl, "phase"=w152:dbl)
                  n371 = call <vilib>:"Basic Function Generator.vi"("offset"=w148, "reset signal"=TRUE, "sampling info"=cluster{"Fs":dbl, "#s":dbl} {"Fs"=1000.0, "#s"=100.0} ("sampling info 4"), "signal type"=w149, "phase"=w152, "amplitude"=w151, "frequency"=w150) -> ("signal out"=w147:waveform(dbl))  [unwired: 2 in, 2 out]
                }
                n372 = Index Array(array=w134) -> (element #1=w138:waveform(dbl), element #2=w137:waveform(dbl), element #3=w136:waveform(dbl), element #4=w135:waveform(dbl))  [unwired: 4 in]
                n373 = property on="Channel 1 Wave (Main)" class="WFGraph (strict)"("Value"=w138) -> ()  [unwired: 2 in, 2 out]
                n374 = property on="Channel 2 Wave (Main)" class="WFGraph (strict)"("Value"=w137) -> ()  [unwired: 2 in, 2 out]
                n375 = property on="Channel 3 Wave (Main)" class="WFGraph (strict)"("Value"=w136) -> ()  [unwired: 2 in, 2 out]
                n376 = property on="Channel 4 Wave (Main)" class="WFGraph (strict)"("Value"=w135) -> ()  [unwired: 2 in, 2 out]
                n377 = call "DAQ Assistant6"("data"=w134, "device name"=tag "cDAQ2Mod1") -> ()  [unwired: 16 in, 2 out]
                n378 = disable-structure shown="Disabled" {
                  frame Disabled {
                    # "daq2"
                    n379 = call "DAQ Assistant4"("device name"=tag "cDAQ3Mod1") -> ()  [unwired: 17 in, 2 out]
                  }
                  frame Enabled {
                  }
                }
              }
              frame "Center" {
                n380 = Unbundle("Center") -> ("Channel 1"=w164:T29, "Channel 2"=w163:T30, "Channel 3"=w162:T30, "Channel 4"=w161:T30)
                n381 = Build Array(w164, w163, w162, w161) -> (w160:T32)
                n382 = for {
                  tunnel: w160 -> [w166] mode=indexing
                  tunnel: [w167] -> w155 mode=indexing
                  n383 = Unbundle By Name(w166) -> ("offset"=w168:i32, "signal type 1"=w169:T19, "frequency 1"=w170:i32, "amplitude 1"=w171:dbl, "phase"=w172:dbl)
                  n384 = call <vilib>:"Basic Function Generator.vi"("offset"=w168, "reset signal"=TRUE, "sampling info"=cluster{"Fs":dbl, "#s":dbl} {"Fs"=1000.0, "#s"=100.0} ("sampling info 4"), "signal type"=w169, "phase"=w172, "amplitude"=w171, "frequency"=w170) -> ("signal out"=w167:waveform(dbl))  [unwired: 2 in, 2 out]
                }
                n385 = Index Array(array=w155) -> (element #1=w159:waveform(dbl), element #2=w158:waveform(dbl), element #3=w157:waveform(dbl), element #4=w156:waveform(dbl))  [unwired: 4 in]
                n386 = property on="Channel 1 Wave (Main)" class="WFGraph (strict)"("Value"=w159) -> ()  [unwired: 2 in, 2 out]
                n387 = property on="Channel 2 Wave (Main)" class="WFGraph (strict)"("Value"=w158) -> ()  [unwired: 2 in, 2 out]
                n388 = property on="Channel 3 Wave (Main)" class="WFGraph (strict)"("Value"=w157) -> ()  [unwired: 2 in, 2 out]
                n389 = property on="Channel 4 Wave (Main)" class="WFGraph (strict)"("Value"=w156) -> ()  [unwired: 2 in, 2 out]
                n390 = call "DAQ Assistant5"("data"=w155) -> ()  [unwired: 17 in, 2 out]
                n391 = disable-structure shown="Disabled" {
                  frame Disabled {
                    # "daq2"
                    n392 = call "DAQ Assistant3"() -> ()  [unwired: 18 in, 2 out]
                  }
                  frame Enabled {
                  }
                }
              }
            }
          }
        }
        n393 = call "FGV_EXIT.vi"("Function"=enum16{"Read", "Write"}."Read") -> ("EXIT out"=w129:bool)  [unwired: 7 in]
      }
    }
    frame #3 {
      n394 = disable-structure shown="RUN_TIME_ENGINE==True" {
        frame condition #0 (active) {
        }
        frame condition #1 {
          n395 = Quit LabVIEW(quit? (T)=TRUE) -> ()
        }
      }
    }
  }
